vi "Mixed Mode Widget.vi"() -> ()   [LabVIEW 2009]
uses:
  lib/MixedMode/Messages/Target.ctl
  lib/Data Access Objects/Metadata/LBCB Number.ctl
  lib/MixedMode/Ramp Time Tuple.ctl
  lib/MixedMode Widget/Mixed Mode State Display.ctl
  lib/MixedMode/Mixed Mode States.ctl
  lib/MixedMode/Messages/Mixed Mode Command.ctl
  lib/MixedMode/Mixed Mode Command Action.ctl
  lib/MixedMode/Target Data.ctl
  lib/MixedMode Widget/Mixed Mode Widget Button States.ctl
  lib/MixedMode Widget/Target Pattern.ctl
  lib/MixedMode/Messages/Mixed Mode Status.ctl
  lib/MixedMode/Mixed Mode Covergance Status.ctl
  lib/MixedMode/Mixed Mode Cartesian Data.ctl
  lib/MixedMode Widget/NTCP MM Requests.ctl
  lib/MixedMode/MCL States.ctl
  lib/MixedMode Widget/Manual States.ctl
  lib/MixedMode Widget/Input File States.ctl
  lib/MixedMode Widget/NTCP Mixed Mode States.ctl
  lib/NTCP Client/NTCP 2 MM Message.ctl
  NTCP library/NTCP Commands.ctl
  lib/MixedMode/Messages/Mixed Mode Button Events Message.ctl
  lib/MixedMode/Messages/Mixed Mode Button Events.ctl
  lib/Apps/GUI Control.ctl
  lib/MixedMode/Messages/MM Widget Parameter Changes.ctl
  lib/MixedMode/Messages/Mixed Mode Gui Update Msg.ctl
  lib/MixedMode/Messages/Mixed Mode GUI Update Type.ctl
  lib/Global Data/Name Actions.ctl
  lib/MixedMode Widget/Blinkies.ctl
  lib/Apps/On Off Button.ctl
  lib/NTCP Client/MM 2 NTCP Message.ctl
  lib/Apps/Yes No Button.ctl
  lib/Apps/App Status Actions.ctl
  lib/Data Access Objects/Metadata/DAO Actions.ctl
  lib/MixedMode/Step DAO Actions.ctl
  lib/MixedMode Widget/Input File Step Actions.ctl
  lib/Launcher/NoPanelAppTypes.ctl
  lib/Launcher/Launcher Actions.ctl
  lib/Data Access Objects/Metadata/Persistant DAO Actions.ctl
  lib/MixedMode Widget/Skip NTCP Close Monitor.ctl
  lib/MixedMode Widget/Run Or Stop Result.ctl
panel:
  out "From Queue":string
  out "To Queue":string
  out "NTCP":T1
  out "MCL States":T5
  out "NTCP MM Requests":T6
  out "Force Limit":bool caption="Force"
  out "Displacement Limit":bool caption="Displacement"
  out "Messages":string
  out "Mixed Mode Status":T7={"LBCB Target"=[], "MixedModeStates"=enum."Idle", "LBCB Convergence"=[], "LBCB Measurements"=[]}
  in  "App Running":bool
  out "Button States":T12
  in  "App Stop":bool
  out "Mixed Mode Command":T13
  in  "Cartesian Type":bool caption="CartesianType"
  in  "Channel Data Tables":T16(tab)
  out "Cartesian Space Labels L1":string[](array[string])=["Commands (in/rad)", "Displacements (in/rad)", "Forces (lbs/lb*in)"]
  out "Cartesian Labels L1":string[](array[string])=["X", "Y", "Z", "Rx", "Ry", "Rz"]
  out "LBCB 1 Cartesian Space":dbl[][](array[numeric]) caption="LBCB 1"
  out "LBCB 2 Cartesian Space":dbl[][](array[numeric]) caption="LBCB 2"
  out "Cartesian Labels L2":string[](array[string])=["X", "Y", "Z", "Rx", "Ry", "Rz"]
  out "Cartesian Space Labels L2":string[](array[string])=["Commands (in/rad)", "Displacements (in/rad)", "Forces (lbs/lb*in)"]
  out "Actuator Space Labels L2":string[](array[string])=["Commands (in)", "Displacements (in)", "Forces (lbs)", "Integral"]
  out "Actuator Labels L2":string[](array[string])=["X1", "X2", "Y1", "Z1", "Z2", "Z3"]
  out "LBCB 2 Actuator Space":dbl[][](array[numeric]) caption="LBCB 2"
  out "LBCB 1 Actuator Space":dbl[][](array[numeric]) caption="LBCB 1"
  out "Actuator Labels L1":string[](array[string])=["X1", "X2", "Y1", "Z1", "Z2", "Z3"]
  out "Actuator Space Labels L1":string[](array[string])=["Commands (in)", "Displacements (in)", "Forces (lbs)", "Integral"]
  out "External Sensors":cluster{"Name":string, "Value":dbl}[](array[cluster])
  out "Test Statistics":cluster{"Steps":string, "Elapsed \nTime":dbl} {"Elapsed \nTime" format="%<%H:%M:%S>t"}
  in  "Mixed Mode Control Tabs":enum32{"Manual", "Input File", "NTCP"}(tab)
  in  "Set Initial Position":bool
  in  "Set Target":bool
  in  "Target Pattern":T17
  in  "Apply Pattern":bool
  out "Manual States":T18
  in  "Run Infile":bool
  out "Running":bool
  in  "Reset":bool
  in  "Load File":bool
  out "Input File States":T19
  in  "Connect Server":bool
  in  "Control Point":string="MDL-00-01"
  out "Connected":bool
  out "NTCP MM States":T20
  in  "Execute":cluster{"Auto":bool, "Start":bool, "Stop":bool}
  in  "Propose":T21
  out "Mixed Mode State Display":T22
  out "Current Values":T3[](array[typedef])
  in  "Ramp Times":cluster{"Displacement":T15, "Force":T15}={"Displacement"={"Ramp"=5.0, "Stab"=4.0, "Hold"=5.0}, "Force"={"Ramp"=5.0, "Stab"=4.0, "Hold"=5.0}}
  in  "Targets":T3[](array[typedef])
  # "Limit\nFaults"
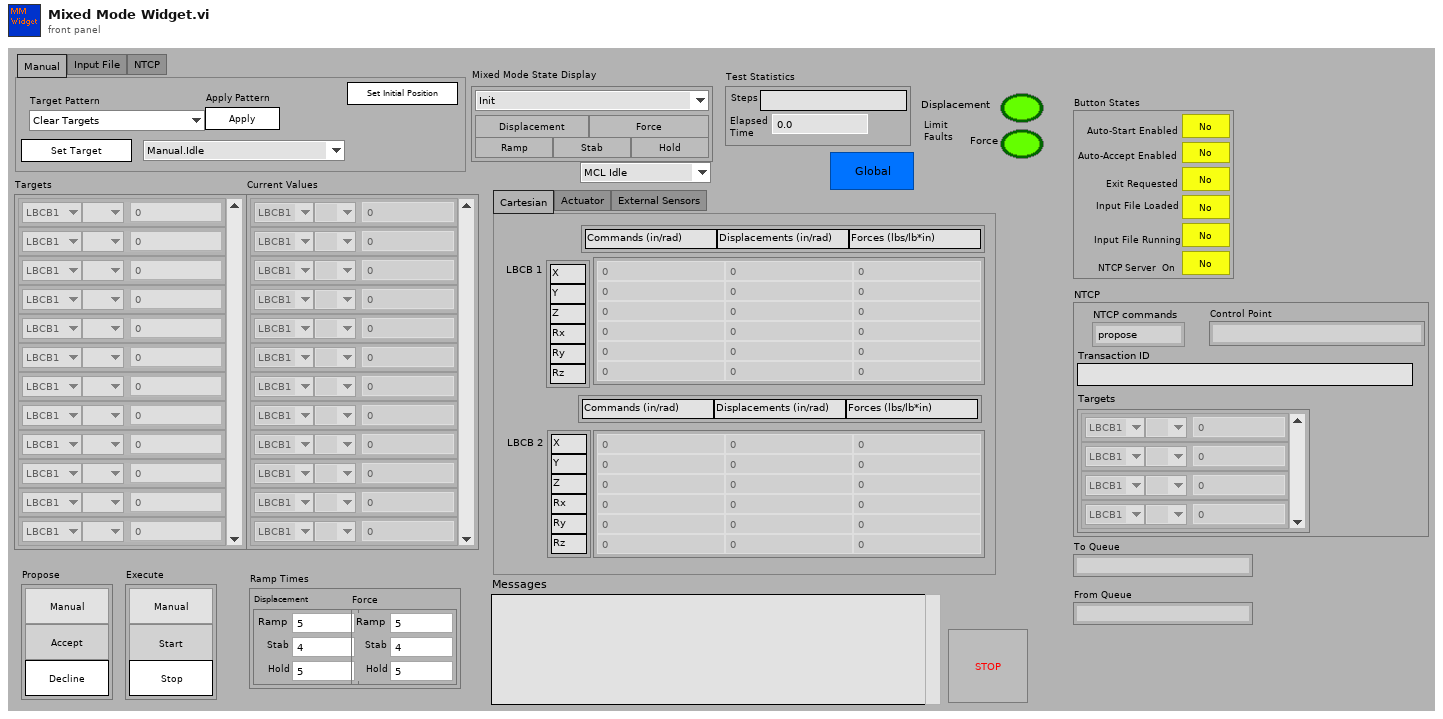
[diagram p1: front panel]
types:
  T1 = typedef "NTCP 2 MM Message.ctl" = cluster{"NTCP commands":T2, "Transaction ID":string, "Control Point":string, "Targets":T3[]}
  T2 = typedef "NTCP Commands.ctl" = enum16{"propose", "execute", "cancel", "set-parameter", "get-parameter", "open-session", "close-session", "get-control-point", "Unknown", "stop"}
  T3 = typedef "Target.ctl" = cluster{"LBCB Number":T4, "DOF Vectors":enum16{" ", "Dx", "Dy", "Dz", "Rx", "Ry", "Rz", "Fx", "Fy", "Fz", "Mx", "My", "Mz"}, "Amount":dbl}
  T4 = typedef "LBCB Number.ctl" = enum16{"LBCB1", "LBCB2"}
  T5 = typedef "MCL States.ctl" = enum16{"MCL Idle", "MCL Ramping", "MCL Holding", "MCL Aborting", "MCL Done", "MCL NOP"}
  T6 = typedef "NTCP MM Requests.ctl" = cluster{"Execute Pending":bool, "Propose Pending":bool, "Connected":bool, "Reset":bool}
  T7 = typedef "Mixed Mode Status.ctl" = cluster{"LBCB Target":T8[], "MixedModeStates":T9, "LBCB Convergence":T10[], "LBCB Measurements":T11[]}
  T8 = typedef "Target Data.ctl" = cluster{"Displacements":dbl[], "Command Type":enum16{"<None>", "Displacement", "Force"}[], "Forces":dbl[]}
  T9 = typedef "Mixed Mode States.ctl" = enum16{"Init", "Wait For DAQ", "Idle", "Start Initial Position", "Initial Position", "Start Initial Ramp", "Run Initial Ramp", "Start Iterative Stage", "Convergence Check", "Update Stiffness Jacobian", "Update Command", "Start Iterative Ramp", "Run Iterative Ramp", "Start Iterative Stabilize", "Iterative Stabilize", "Start Iterative Holding", "Iterative Holding", "Start Stabilize", "Stabilize", "Start Hold", "Holding", "Done", "Aborting", "Exit", "Nop"}
  T10 = typedef "Mixed Mode Covergance Status.ctl" = cluster{"IsConverged":bool[], "Force Errors":dbl[], "Controlling DOF":bool[]}
  T11 = typedef "Mixed Mode Cartesian Data.ctl" = cluster{"Displacements":dbl[], "Forces":dbl[]}
  T12 = typedef "Mixed Mode Widget Button States.ctl" = cluster{"Auto-Start Enabled":bool, "Auto-Accept Enabled":bool, "Exit Requested":bool, "Input File Loaded":bool, "Input File Running":bool, "NTCP Server  On":bool}
  T13 = typedef "Mixed Mode Command.ctl" = cluster{"Command":T14, "Ramp Times":cluster{"Initial":T15, "Iterative":T15}, "LBCB1":T8, "LBCB2":T8}
  T14 = typedef "Mixed Mode Command Action.ctl" = enum16{"Start Command", "Stop", "Exit", "No Op", "Start Acquisition", "Measure Initial Position"}
  T15 = typedef "Ramp Time Tuple.ctl" = cluster{"Ramp":dbl, "Stab":dbl, "Hold":dbl}
  T16 = enum32{"Cartesian", "Actuator", "External Sensors"}
  T17 = typedef "Target Pattern.ctl" = enum16{"Clear Targets", "Reset Targets to Zero", "Displacements Only", "Rotations Only", "Displacements & Rotations", "Forces Only", "Moments Only", "Forces & Moments"}
  T18 = typedef "Manual States.ctl" = enum16{"Manual.Idle", "Manual.WaitForStart", "Manual.WaitForMclRamp", "Manual.WaitForMclDone", "Manual.Abort", "Manual.InitialPosition"}
  T19 = typedef "Input File States.ctl" = enum16{"InputFile.Idle", "InputFile.WaitForRunning", "InputFile.StepsAvailable", "InputFile.LoadStep", "InputFile.WaitForAccept", "InputFile.WaitForStart", "InputFile.WaitForMclRamp", "InputFile.WaitForMclDone", "InputFile.StopRunning"}
  T20 = typedef "NTCP Mixed Mode States.ctl" = enum16{"Ntcp.Off", "Ntcp.WaitForProposal", "Ntcp.WaitForAccept", "Ntcp.WaitForExecute", "Ntcp.WaitForStart", "Ntcp.WaitForMclRamp", "Ntcp.WaitForMclDone", "Ntcp.Shutdown"}
  T21 = cluster{"Auto":bool, "Accept":bool, "Decline":bool}
  T22 = typedef "Mixed Mode State Display.ctl" = cluster{"MixedModeStates":T9, "Initial":bool, "Iterative":bool, "Ramp":bool, "Stab":bool, "Hold":bool}
  T23 = typedef "MM 2 NTCP Message.ctl" = cluster{"NTCP commands":T2, "Transaction ID":string, "Control Point":string, "Accepted":T24}
  T24 = typedef "Yes No Button.ctl" = bool
  T25 = typedef "Blinkies.ctl" = cluster{"Accept":T26, "Start":T26}
  T26 = typedef "On Off Button.ctl" = bool
  T27 = typedef "Name Actions.ctl" = enum16{"Init", "Get Names", "Get Index"}
  T28 = typedef "Mixed Mode Gui Update Msg.ctl" = cluster{"MM GUI Update Type":T29, "Targets":T3[], "State":bool, "Step":string}
  T29 = typedef "Mixed Mode GUI Update Type.ctl" = enum16{"Nop", "Targets", "Accept.Blink", "Start.Blink", "TestStats", "Control.Enabled", "StartTestTimer", "RunInputFile", "NTCP Server", "Propose.Auto", "Execute.Auto", "All Autos Off", "Input File Loaded", "Exit"}
  T30 = typedef "GUI Control.ctl" = cluster{"Command":T31, "LBCB Number":enum16{"LBCB1", "LBCB2"}}
  T31 = typedef "MM Widget Parameter Changes.ctl" = enum16{"Start", "Stop All", "Cartesian Type Changed", "Control Enabled", "Control Disabled", "NTCP Link On", "NTCP Link Off"}
  T32 = typedef "Mixed Mode Button Events Message.ctl" = cluster{"MM Control Events":T33, "Button States":T12}
  T33 = typedef "Mixed Mode Button Events.ctl" = enum16{"Propose.Accept", "Propose.Decline", "Execute.Start", "Execute.Stop", "TargetSet", "InputFile.Load", "InputFile.Reset", "InputFile.Pause", "InputFile.Run", "CartesianType.Changed", "NCTP.ConnectToServer", "NTCP.DisconnectFromServer", "Application.Stop", "Control.Enabled", "Control.Disabled", "ControlType.Changed", "Nop", "Manual.SetInitialPosition"}
  T34 = typedef "DAO Actions.ctl" = enum16{"Init", "Get", "Set"}
  T35 = typedef "App Status Actions.ctl" = enum16{"Init", "Get Status", "Running", "Control", "Autobalanced", "Data Acquisition", "Set App State", "DAQ Started", "Set LBCB State", "Set All", "Set Cont Logging", "Set Step Logging", "Set MM Logging", "Set Volt Logging", "Set Cart Type", "Set DAQ Link", "Set NTCP Link"}
  T36 = typedef "Step DAO Actions.ctl" = enum16{"Init", "Set", "Get", "Reset Count"}
  T37 = typedef "App Status.ctl" = cluster{"Running":bool, "Controlling L2":bool, "Autobalance L2":bool, "Data Acquisition":bool, " App State":T38, "DAQ Started":bool, "LBCB 1 State":T39, "LBCB 2 State":T39, "Controlling L1":bool, "Autobalance L1":bool, "Cartesian Type":bool, "Continuous Logging":bool, "Step Logging":bool, "Voltage Logging":bool, "Mixed Mode Logging":bool, "DAQ Link":bool, "NTCP Link ":bool}
  T38 = typedef "AppStates.ctl" = enum16{"Starting OM", "Initializing Displays", "Setting up Archiving", "Setting Up DAQ Channels", "Start DAQ", "DAQ Starting", "Controlling LBCBs", "Stopping OM"}
  T39 = typedef "Lbcb Control Loop States.ctl" = enum16{"Idle", "Start Selected", "Load Last Command", "Start Autobalancing", "Autobalancing", "Control Loop Initialized", "Control Enabled"}
  T40 = enum8{"Enabled", "Disabled", "Disabled and Grayed Out"}
  T41 = typedef "Input File Step Actions.ctl" = enum16{"Load", "Next Step", "Reset", "Get Step", "Backup"}
  T42 = typedef "Run Or Stop Result.ctl" = enum16{"Nevermind", "Run", "Stop"}
  T43 = typedef "Load Step.ctl" = cluster{"Step Number":u32, "Targets":T3[]}
  T44 = typedef "Accepted or Declined.ctl" = enum16{"No Decision Yet", "Accepted", "Declined", "Abort"}
  T45 = typedef "Stop Requests.ctl" = enum16{"Nothing", "Stop Requested", "Abort Requested"}
  T46 = typedef "MCL Done Or Abort.ctl" = enum16{"Done", "Abort", "Still Running"}
  T47 = typedef "NoPanelAppTypes.ctl" = enum16{"NTCP Socket", "Data Archiving", "DAQ Link", "Control Loops", "Autobalance Monitor", "Mixed Mode Monitor", "Cmd Disp Diffs"}
  T48 = typedef "Launcher Actions.ctl" = enum16{"Launch", "Stop All", "Stop", "Kill", "Running?", "Init"}
  T49 = typedef "Persistant DAO Actions.ctl" = enum16{"Init", "Get", "Set", "Load", "Save"}
  T50 = typedef "Skip NTCP Close Monitor.ctl" = enum16{"Skip Nothing", "Skip NTCP", "Skip Button Event"}
  T51 = typedef "Network Parameters.ctl" = cluster{"Port Number":u16, "Notification Name":string, "Wait For Notification Timeout":i32}
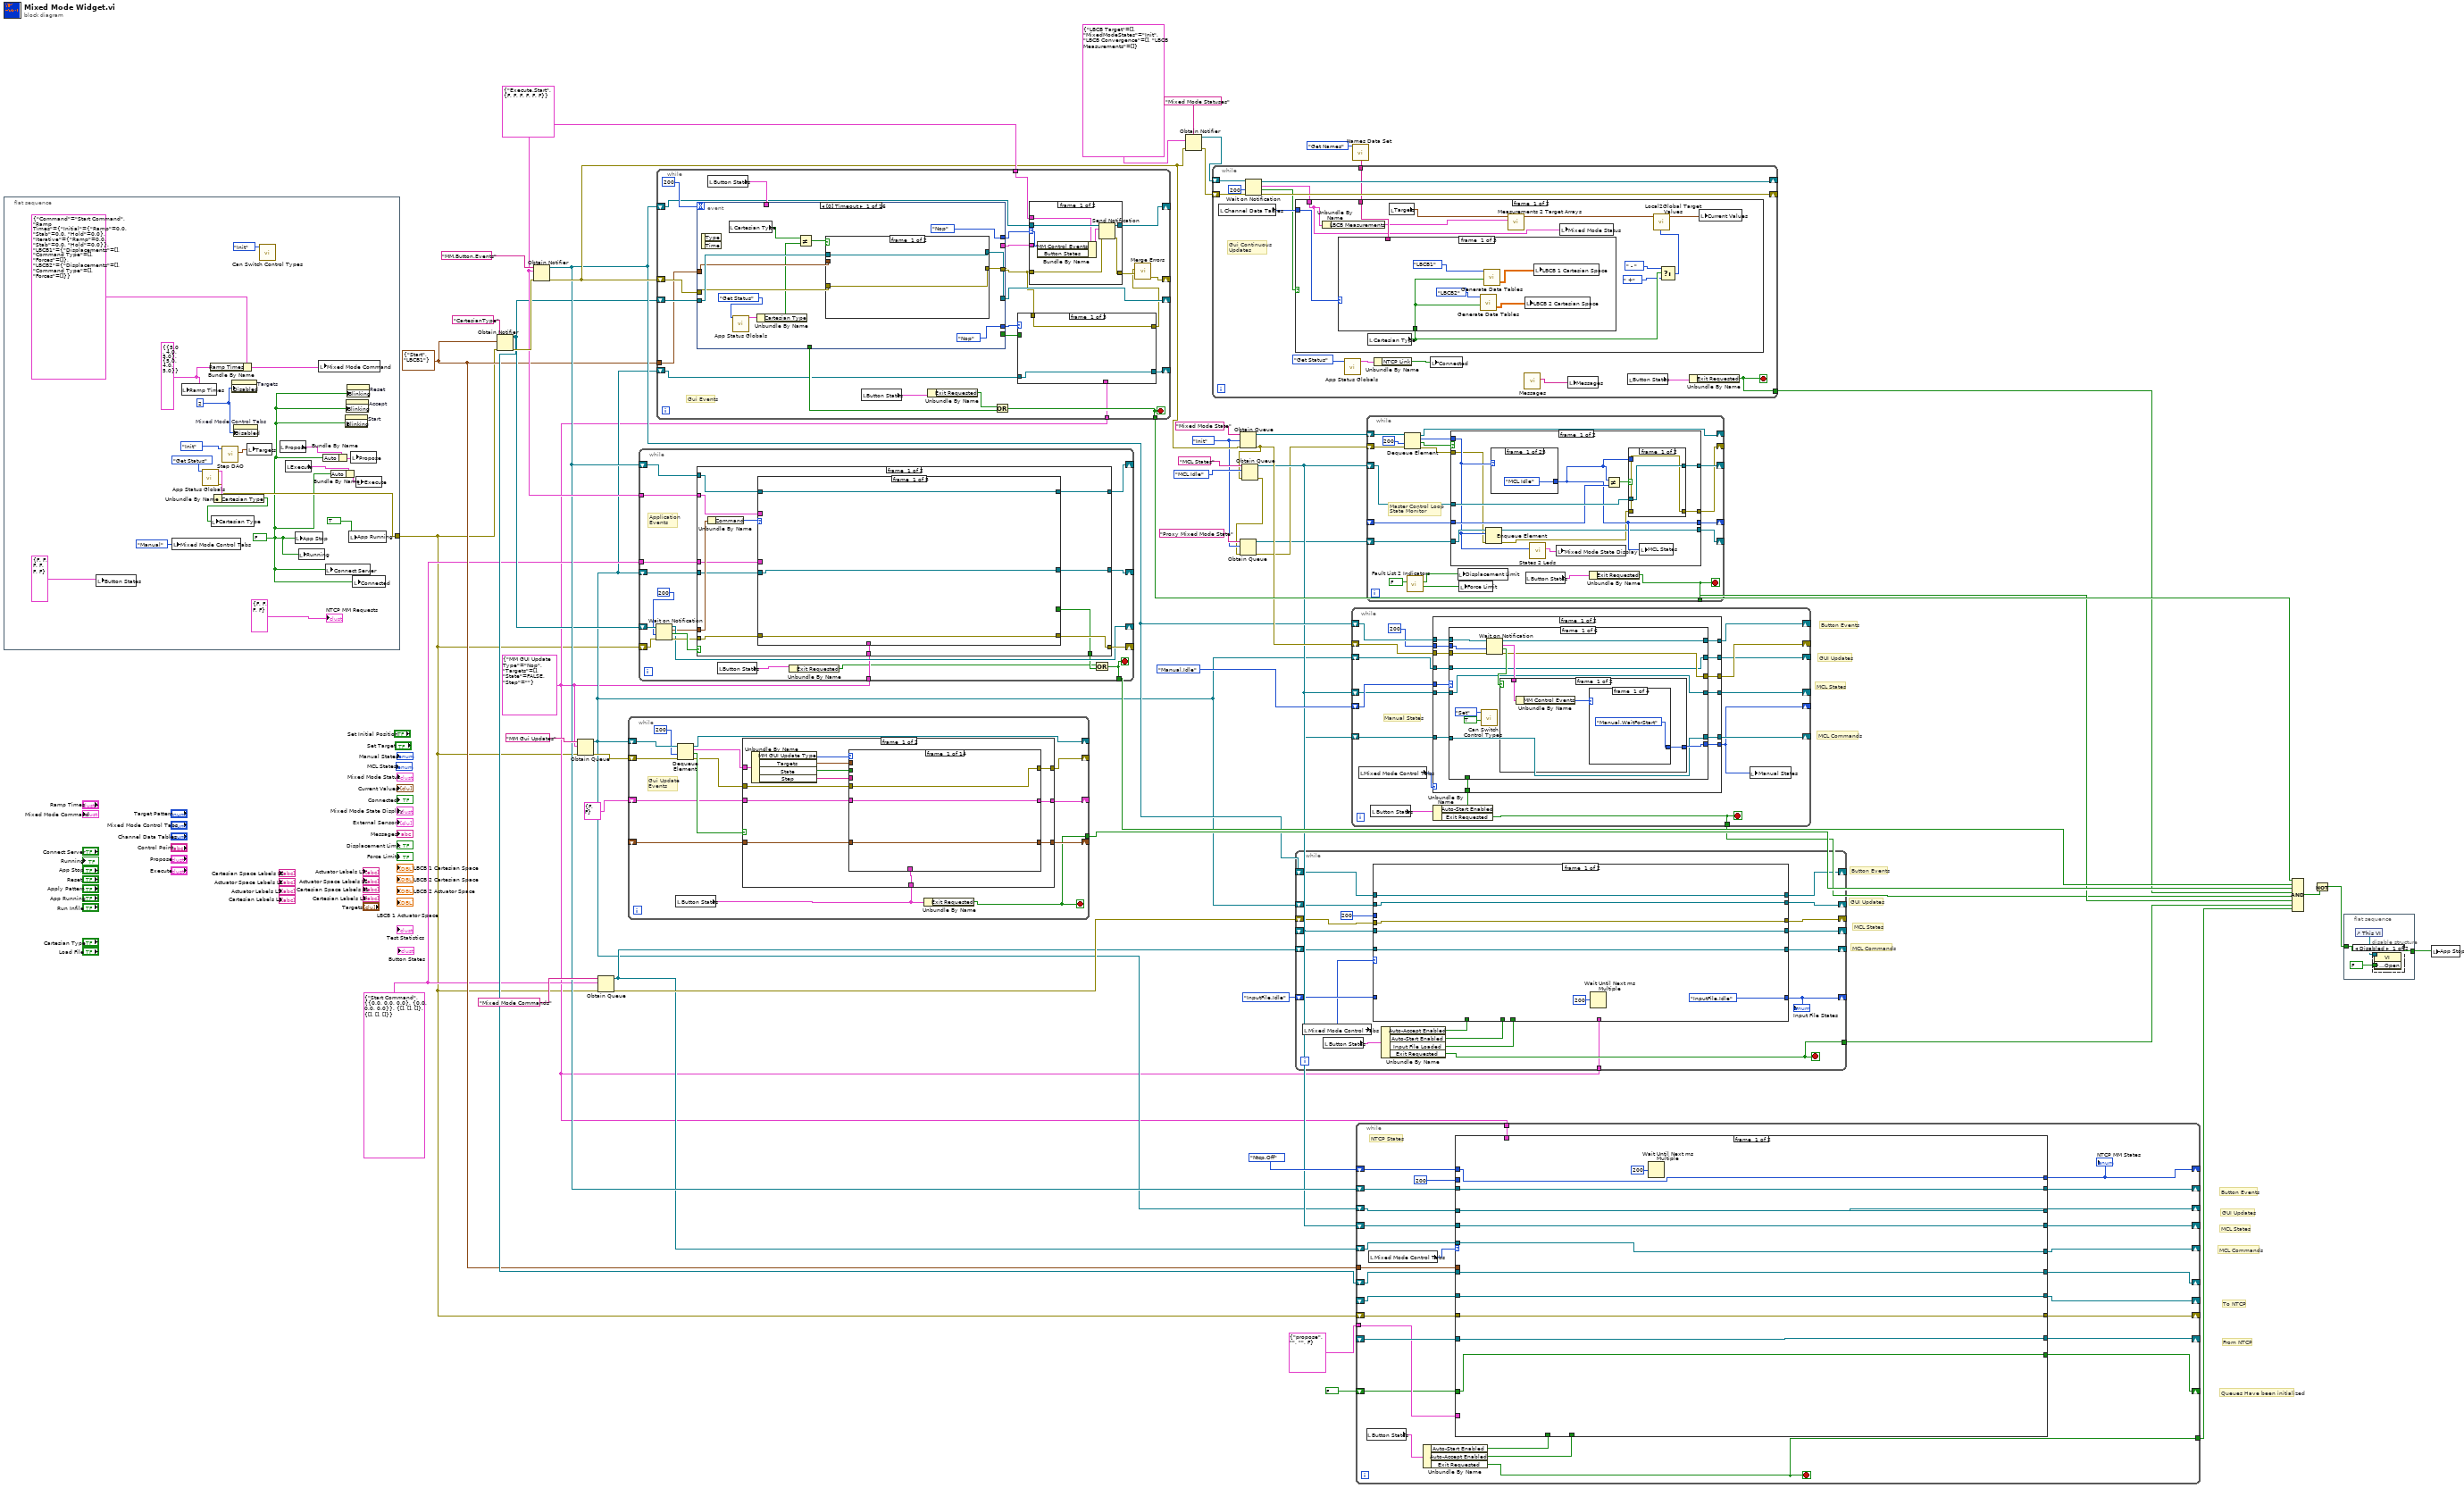
[diagram p0: block diagram]
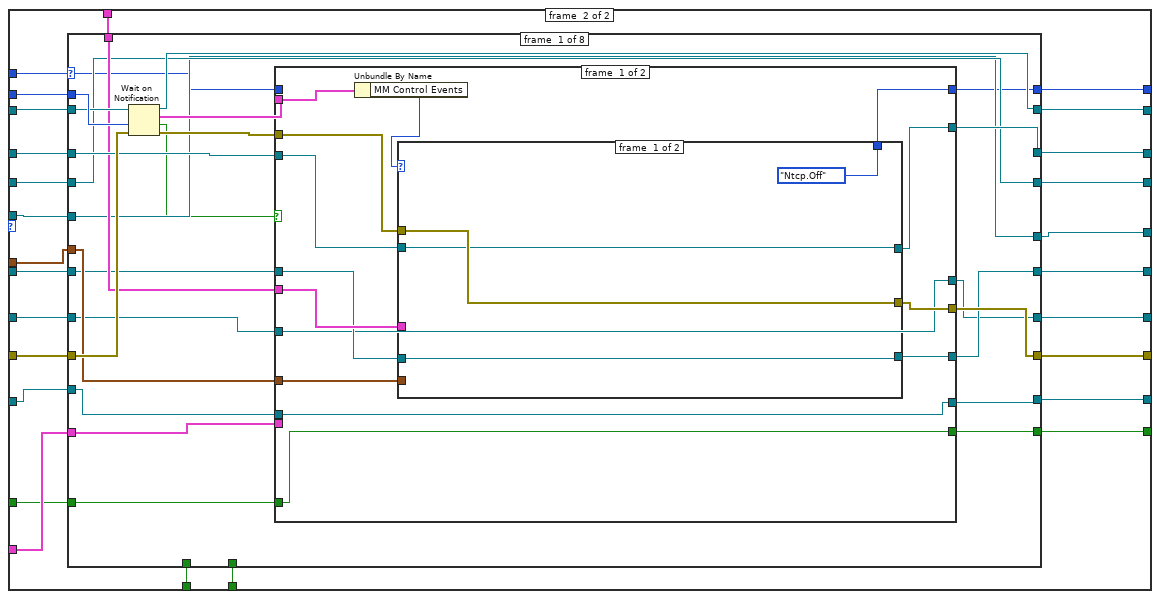
[diagram p2: hidden frame]
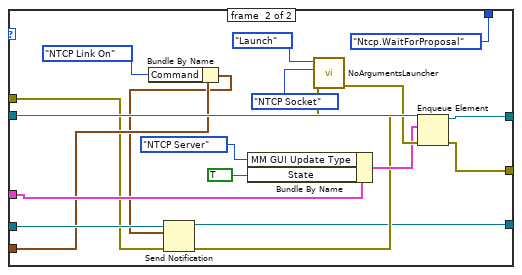
[diagram p3: hidden frame]
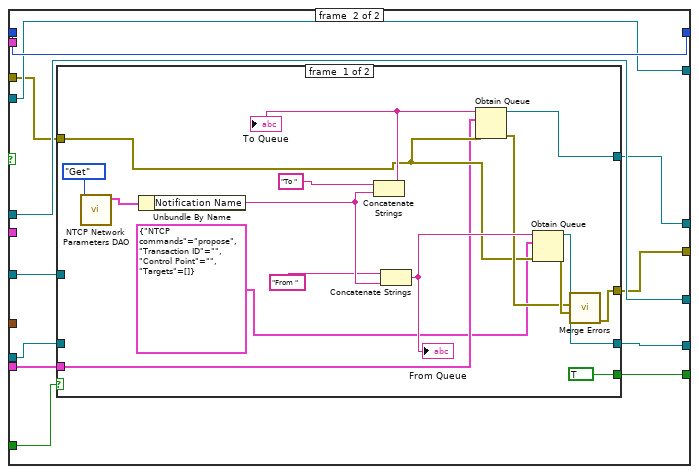
[diagram p4: hidden frame]
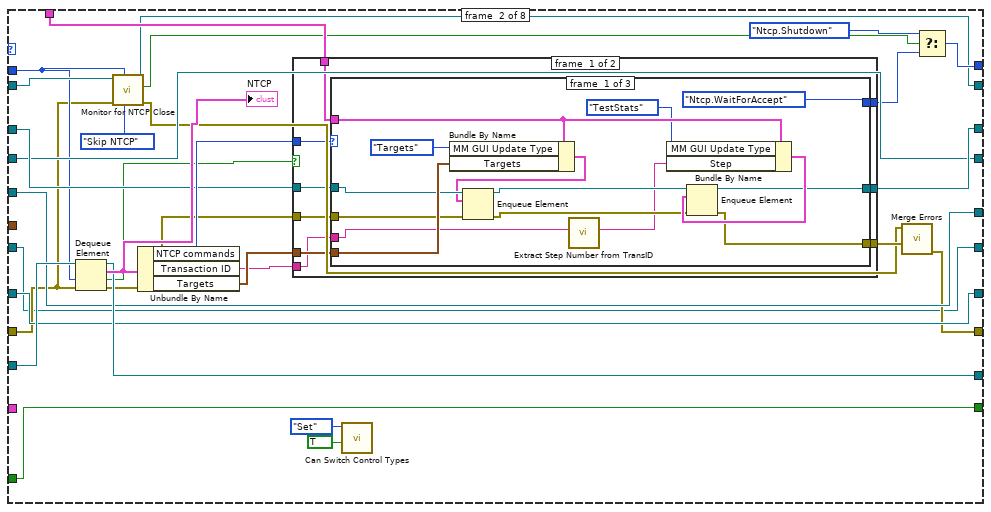
[diagram p6: hidden frame]
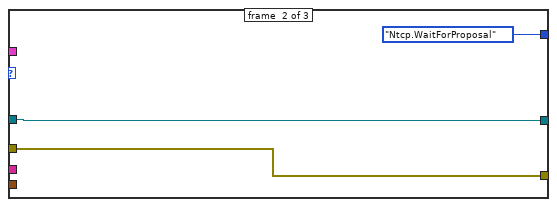
[diagram p7: hidden frame]
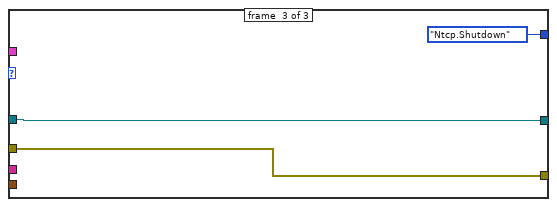
[diagram p8: hidden frame]
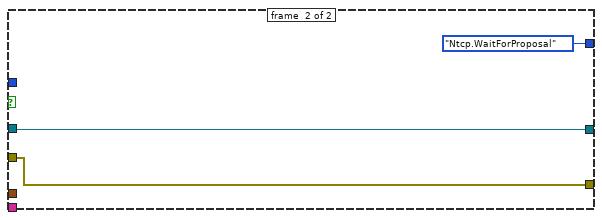
[diagram p9: hidden frame]
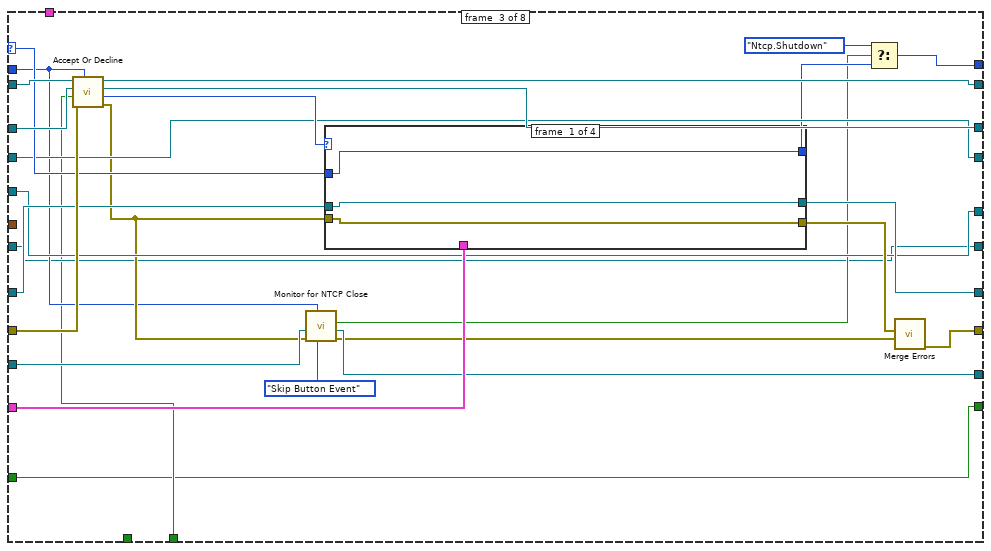
[diagram p10: hidden frame]
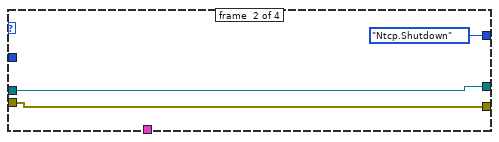
[diagram p11: hidden frame]
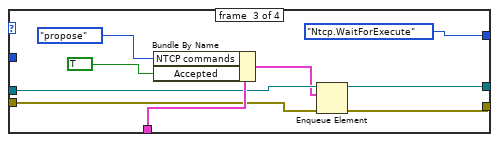
[diagram p12: hidden frame]
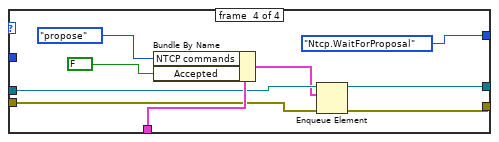
[diagram p13: hidden frame]
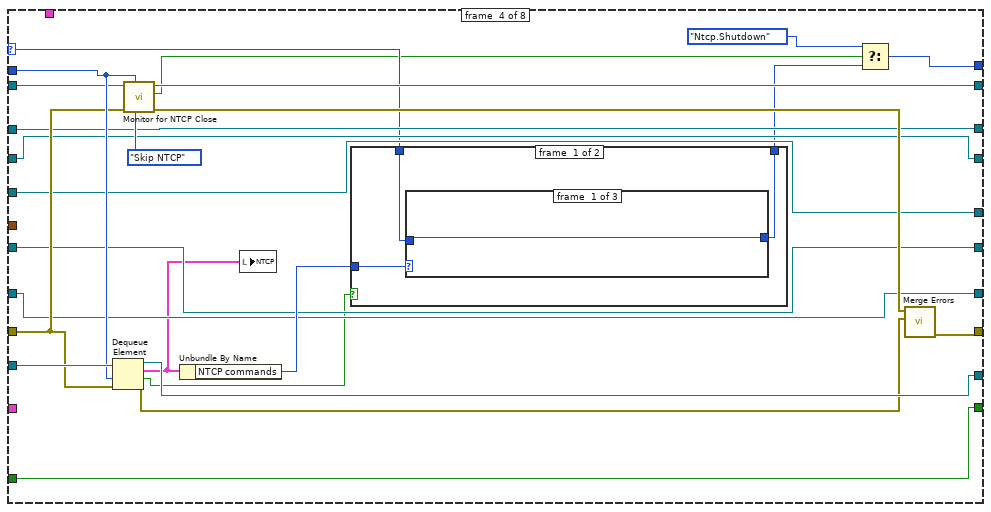
[diagram p14: hidden frame]
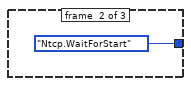
[diagram p15: hidden frame]
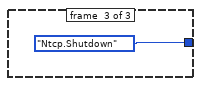
[diagram p16: hidden frame]
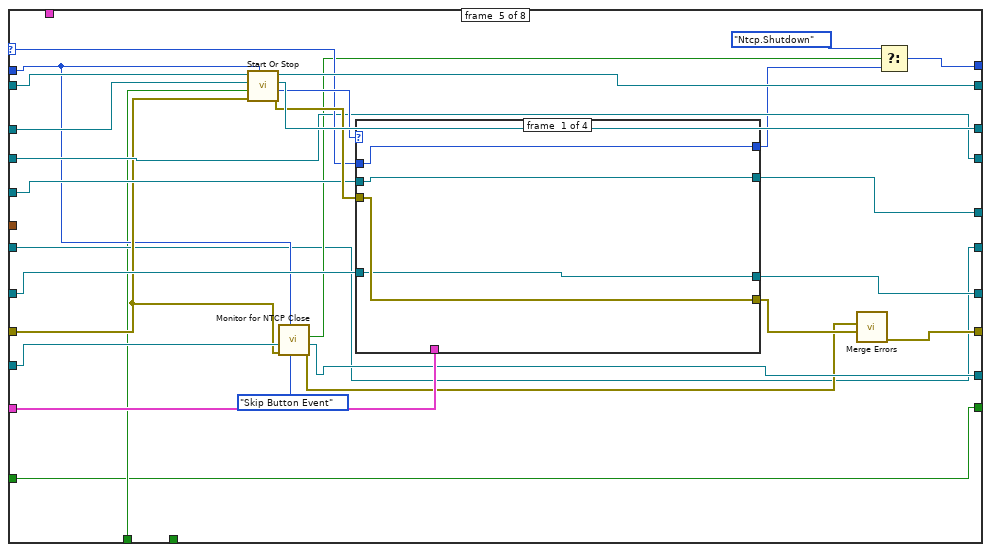
[diagram p18: hidden frame]
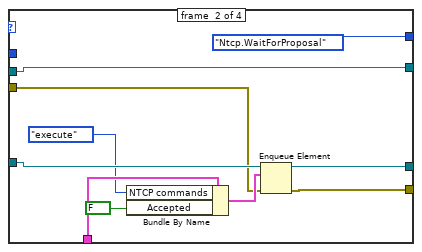
[diagram p19: hidden frame]
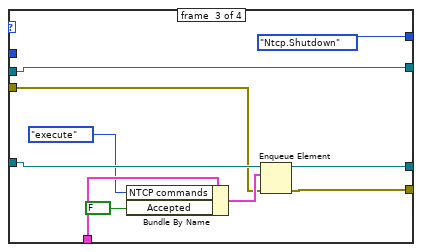
[diagram p20: hidden frame]
diagram:
  w12 = T13 {"Command"=enum."Start Command", "Ramp Times"={"Initial"={"Ramp"=0.0, "Stab"=0.0, "Hold"=0.0}, "Iterative"={"Ramp"=0.0, "Stab"=0.0, "Hold"=0.0}}, "LBCB1"={"Displacements"=[], "Command Type"=[], "Forces"=[]}, "LBCB2"={"Displacements"=[], "Command Type"=[], "Forces"=[]}} ("Mixed Mode Command In")
  w4 = Mixed_Mode_States."Init" ("f")
  w9 = T28 {"MM GUI Update Type"=enum."Nop", "Targets"=[], "State"=FALSE, "Step"=""} ("MM Gui Update Msg")
  w14 = T30 {"Command"=enum."Start", "LBCB Number"=enum."LBCB1"} ("GUI Control")
  w45 = T32 {"MM Control Events"=enum."Execute.Start", "Button States"={"Auto-Start Enabled"=FALSE, "Auto-Accept Enabled"=FALSE, "Exit Requested"=FALSE, "Input File Loaded"=FALSE, "Input File Running"=FALSE, "NTCP Server  On"=FALSE}} ("MM Button Events Msg")
  # "Queues Have been initialized"
  # "Button Events"
  # "GUI Updates"
  # "MCL States"
  # "MCL Commands"
  # "From NTCP"
  # "To NTCP"
  # "Button Events"
  # "GUI Updates"
  # "MCL States"
  # "MCL Commands"
  # "Button Events"
  # "GUI Updates"
  # "MCL States"
  # "MCL Commands"
  n1 = flat-sequence {
    tunnel: [w69] -> w8
    frame #0 {
      w58 = cluster{"Initial":T15, "Iterative":T15} {"Initial"={"Ramp"=5.0, "Stab"=4.0, "Hold"=5.0}, "Iterative"={"Ramp"=5.0, "Stab"=4.0, "Hold"=5.0}} ("Ramp Times")
      w59 = u8 2 ("Disabled")
      w53 = FALSE ("Exit")
      n2 = local write "Button States"(T12 {"Auto-Start Enabled"=FALSE, "Auto-Accept Enabled"=FALSE, "Exit Requested"=FALSE, "Input File Loaded"=FALSE, "Input File Running"=FALSE, "NTCP Server  On"=FALSE} ("Mixed Mode Widget Requests")) -> ()
      n3 = local write "Mixed Mode Control Tabs"(enum32{"Manual", "Input File", "NTCP"}."Manual" ("Mixed Mode Control Tabs")) -> ()
      n4 = local write "Ramp Times"(w58) -> ()
      n5 = call "App Status Globals.vi"("App Status Actions"=App_Status_Actions."Get Status") -> ("App Status Out"=w71:T37, "error out"=w69:errorcluster)  [unwired: 5 in, 8 out]
      n6 = Bundle By Name(cluster=T13 {"Command"=enum."Start Command", "Ramp Times"={"Initial"={"Ramp"=0.0, "Stab"=0.0, "Hold"=0.0}, "Iterative"={"Ramp"=0.0, "Stab"=0.0, "Hold"=0.0}}, "LBCB1"={"Displacements"=[], "Command Type"=[], "Forces"=[]}, "LBCB2"={"Displacements"=[], "Command Type"=[], "Forces"=[]}} ("Mixed Mode Command"), "Ramp Times"=w58) -> (w56:T13)
      n7 = Unbundle By Name(w71) -> ("Cartesian Type"=w70:bool)
      n8 = local write "Cartesian Type"(w70) -> ()
      n9 = call "Step DAO.vi"("Step DAO Actions"=Step_DAO_Actions."Init") -> ("Step Out"=w67:T3[])  [unwired: 3 in, 7 out]
      n10 = property on="Targets" class="Arr (strict)"("Disabled"=w59) -> ()  [unwired: 2 in, 2 out]
      n11 = property on="Mixed Mode Control Tabs" class="TabCtl (strict)"("Disabled"=w59) -> ()  [unwired: 2 in, 2 out]
      n12 = local write "Targets"(w67) -> ()
      n13 = call "Can Switch Control Types.vi"("DAO Actions"=DAO_Actions."Init") -> ()  [unwired: 10 in, 1 out]
      n14 = local read "Propose"() -> (w63:T21)
      n15 = local read "Execute"() -> (w61:cluster{"Auto":bool, "Start":bool, "Stop":bool})
      n16 = local write "App Stop"(w53) -> ()
      n17 = local write "Running"(w53) -> ()
      n18 = local write "Mixed Mode Command"(w56) -> ()
      n19 = Bundle By Name(cluster=w63, "Auto"=w53) -> (w64:T21)
      n20 = local write "Connect Server"(w53) -> ()
      n21 = Bundle By Name(cluster=w61, "Auto"=w53) -> (w62:cluster{"Auto":bool, "Start":bool, "Stop":bool})
      n22 = property on="Start" class="Bool (strict)"("Blinking"=w53) -> ()  [unwired: 2 in, 2 out]
      n23 = property on="Accept" class="Bool (strict)"("Blinking"=w53) -> ()  [unwired: 2 in, 2 out]
      n24 = property on="Reset" class="Bool"("Blinking"=w53) -> ()  [unwired: 2 in, 2 out]
      n25 = local write "App Running"(TRUE) -> ()
      n26 = local write "Propose"(w64) -> ()
      n27 = local write "Connected"(w53) -> ()
      n28 = local write "Execute"(w62) -> ()
      "NTCP MM Requests" <- T6 {"Execute Pending"=FALSE, "Propose Pending"=FALSE, "Connected"=FALSE, "Reset"=FALSE} ("NTCP MM Requests")
    }
  }
  n29 = Obtain Notifier(name (unnamed)="CartesianType", notification data type=w14, error in (no error)=w8) -> (notifier out=w15:refnum<notifier>, error out=w46:errorcluster)  [unwired: 1 in, 1 out]
  n30 = Obtain Notifier(name (unnamed)="MM.Button.Events", notification data type=w45, error in (no error)=w46) -> (notifier out=w18:refnum<notifier>, error out=w31:errorcluster)  [unwired: 1 in, 1 out]
  n31 = Obtain Queue(name (unnamed)="MM Gui Updates", element data type=w9, error in (no error)=w8) -> (queue out=w11:refnum<queue>, error out=w41:errorcluster)  [unwired: 2 in, 1 out]
  n32 = Obtain Queue(name (unnamed)="Mixed Mode Commands", element data type=w12, error in (no error)=w8) -> (queue out=w13:refnum<queue>, error out=w20:errorcluster)  [unwired: 2 in, 1 out]
  n33 = while {
    shift-right: [w78] -> _
    shift-left: w41 -> [w83]
    shift-right: [w82] -> _
    shift-left: w11 -> [w85]
    shift-right: [w77] -> _
    shift-left: _ -> [w76]
    tunnel: [w75] -> w40
    shift-right: [w72] -> _
    shift-left: T25 {"Accept"=FALSE, "Start"=FALSE} ("Blinkies") -> [w73]
    stop <- w75 stop-if-true
    # "Gui Update\nEvents"
    n34 = local read "Button States"() -> (w74:T12)
    n35 = Dequeue Element(queue=w85, timeout in ms (-1)=200, error in (no error)=w83) -> (queue out=w82:refnum<queue>, element=w81:T28, timed out?=w80:bool, error out=w79:errorcluster)
    n36 = case shown="True" w80 {
      tunnel: w81 -> [w97 _]
      tunnel: w79 -> [w93 w194]
      tunnel: [w92 w194] -> w78
      tunnel: [w90 w193] -> w77
      tunnel: w76 -> [w89 w193]
      tunnel: w74 -> [w88 _]
      tunnel: w73 -> [w87 w192]
      tunnel: [w86 w192] -> w72
      frame #0 {
        n37 = Unbundle By Name(w97) -> ("MM GUI Update Type"=w96:T29, "Targets"=w95:T3[], "State"=w94:bool, "Step"=w91:string)
        n38 = case shown="\"Exit\"" w96 {
          tunnel: w95 -> [_ _ w107 _ _ _ _ _ _ _ _ _ _ _]
          tunnel: w94 -> [_ _ _ w109 w121 _ w141 w147 w154 _ w170 w175 w184 _]
          tunnel: w93 -> [w100 w103 w105 w115 w127 w133 w145 w151 w157 w163 w168 w174 w182 w190]
          tunnel: [w100 w103 w105 w114 w126 w133 w145 w151 w157 w163 w166 w174 w182 w190] -> w92
          tunnel: w91 -> [_ _ _ _ _ w137 _ _ _ _ _ _ _ _]
          tunnel: [w99 w102 w106 w113 w125 w134 w143 w149 w152 w159 w165 w179 w187 w191] -> w90
          tunnel: w89 -> [w99 w102 w106 w113 w125 w134 _ _ w152 w159 w165 w179 w187 _]
          tunnel: w88 -> [_ _ _ _ _ _ w142 w148 w155 w161 _ w178 w186 _]
          tunnel: w87 -> [w98 w101 w104 w110 w122 w132 w144 w150 w156 w162 w164 w173 w181 w189]
          tunnel: [w98 w101 w104 w108 w120 w132 w144 w150 w156 w162 w164 w173 w181 w189] -> w86
          frame #0 {
          }
          frame #1 {
          }
          frame #2 {
            n39 = local write "Targets"(w107) -> ()
          }
          frame #3 {
            n40 = Unbundle By Name(w110) -> ("Start"=w111:T26)
            n41 = Not Equal?(x=w109, y=w111) -> (x != y?=w112:T26)
            n42 = case shown="False" w112 {
              tunnel: w115 -> [w116 w119]
              tunnel: w109 -> [_ w118]
              tunnel: [w116 w117] -> w114
              frame #0 {
              }
              frame #1 {
                n43 = property on="Start" class="Bool (strict)"(error in=w119, "Blinking"=w118) -> (error out=w117:errorcluster)  [unwired: 1 in, 1 out]
              }
            }
            n44 = Bundle By Name(cluster=w110, "Start"=w109) -> (w108:T25)
          }
          frame #4 {
            n45 = Unbundle By Name(w122) -> ("Accept"=w123:T26)
            n46 = Not Equal?(x=w121, y=w123) -> (x != y?=w124:T26)
            n47 = case shown="True" w124 {
              tunnel: w127 -> [w128 w131]
              tunnel: w121 -> [_ w130]
              tunnel: [w128 w129] -> w126
              frame #0 {
              }
              frame #1 {
                n48 = property on="Accept" class="Bool (strict)"(error in=w131, "Blinking"=w130) -> (error out=w129:errorcluster)  [unwired: 1 in, 1 out]
              }
            }
            n49 = Bundle By Name(cluster=w122, "Accept"=w121) -> (w120:T25)
          }
          frame #5 {
            n50 = Get Date/Time In Seconds() -> (seconds since 1Jan1904=w135:timestamp)
            n51 = Subtract(x=w135, y=w134) -> (x-y=w136:dbl)
            n52 = Bundle By Name(cluster=cluster{"Steps":string, "Elapsed \nTime":dbl} {"Steps"="", "Elapsed \nTime"=0.0} ("Test Statistics"), "Steps"=w137, "Elapsed \nTime"=w136) -> (w138:cluster{"Steps":string, "Elapsed \nTime":dbl})
            n53 = local write "Test Statistics"(w138) -> ()
          }
          frame #6 {
            n54 = Bundle By Name(cluster=w142, "Input File Running"=w141) -> (w140:T12)
            n55 = local write "Running"(w141) -> ()
            n56 = local write "Button States"(w140) -> ()
            n57 = Get Date/Time In Seconds() -> (seconds since 1Jan1904=w143:timestamp)
          }
          frame #7 {
            n58 = Bundle By Name(cluster=w148, "NTCP Server  On"=w147) -> (w146:T12)
            n59 = local write "Connect Server"(w147) -> ()
            n60 = local write "Button States"(w146) -> ()
            n61 = Get Date/Time In Seconds() -> (seconds since 1Jan1904=w149:timestamp)
          }
          frame #8 {
            n62 = Bundle By Name(cluster=w155, "Input File Loaded"=w154) -> (w153:T12)
            n63 = local write "Button States"(w153) -> ()
          }
          frame #9 {
            n64 = Bundle By Name(cluster=w161, "Exit Requested"=TRUE) -> (w160:T12)
            n65 = local write "Button States"(w160) -> ()
          }
          frame #10 {
            n66 = Select(t=T40."Enabled" ("Disabled"), s=w170, f=T40."Disabled and Grayed Out" ("Disabled")) -> (s? t:f=w169:T40)
            n67 = property on="Mixed Mode Control Tabs" class="TabCtl (strict)"(error in=w168, "DisabledEnum"=w169) -> (error out=w167:errorcluster)  [unwired: 1 in, 1 out]
            n68 = property on="Targets" class="Arr (strict)"(error in=w167, "DisabledEnum"=w169) -> (error out=w166:errorcluster)  [unwired: 1 in, 1 out]
          }
          frame #11 {
            n69 = Bundle By Name(cluster=w178, "Auto-Accept Enabled"=w175) -> (w177:T12)
            n70 = Bundle By Name(cluster=T21 {"Auto"=FALSE, "Accept"=FALSE, "Decline"=FALSE} ("Propose"), "Auto"=w175) -> (w176:T21)
            n71 = local write "Button States"(w177) -> ()
            n72 = local write "Propose"(w176) -> ()
          }
          frame #12 {
            n73 = Bundle By Name(cluster=w186, "Auto-Start Enabled"=w184) -> (w185:T12)
            n74 = Bundle By Name(cluster=T21 {"Auto"=FALSE, "Accept"=FALSE, "Decline"=FALSE} ("Propose"), "Auto"=w184) -> (w183:T21)
            n75 = local write "Button States"(w185) -> ()
            n76 = local write "Execute"(w183) -> ()
          }
          frame #13 {
            n77 = Get Date/Time In Seconds() -> (seconds since 1Jan1904=w191:timestamp)
          }
        }
      }
      frame #1 {
      }
    }
    n78 = Unbundle By Name(w74) -> ("Exit Requested"=w75:bool)
  }
  n79 = while {
    shift-right: [w203] -> _
    shift-left: w18 -> [w205]
    shift-right: [w208] -> _
    shift-left: w15 -> [w212]
    shift-right: [w209] -> _
    shift-left: w8 -> [w211]
    tunnel: w45 -> [w204]
    tunnel: [w197] -> w43
    shift-right: [w199] -> _
    shift-left: w11 -> [w201]
    tunnel: w9 -> [w200]
    tunnel: w12 -> [w195]
    stop <- w197 stop-if-true
    # "Application\nEvents"
    n80 = Wait on Notification(notifier=w212, timeout in ms (-1)=200, error in (no error)=w211) -> (notifier out=w208:refnum<notifier>, notification=w207:T30, timed out?=w213:bool, error out=w210:errorcluster)  [unwired: 1 in]
    n81 = case shown="True" w213 {
      tunnel: w210 -> [w220 w285]
      tunnel: [w219 w285] -> w209
      tunnel: w207 -> [w225 _]
      tunnel: w205 -> [w222 w284]
      tunnel: w204 -> [w223 _]
      tunnel: [w221 w284] -> w203
      tunnel: [w218 _] -> w202
      tunnel: w201 -> [w217 w283]
      tunnel: w200 -> [w216 _]
      tunnel: [w215 w283] -> w199
      tunnel: w195 -> [w214 _]
      frame #0 {
        n82 = Unbundle By Name(w225) -> ("Command"=w224:T31)
        n83 = case shown="\"Control Enabled\"" w224 {
          tunnel: w223 -> [_ w242 w260 w274 w282]
          tunnel: w222 -> [w228 w237 w256 w269 w276]
          tunnel: [w228 w238 w257 w270 w277] -> w221
          tunnel: w220 -> [w227 w239 w248 w261 w279]
          tunnel: [w227 w234 w244 w271 w278] -> w219
          tunnel: [_ w236 _ _ _] -> w218
          tunnel: w217 -> [w226 w232 w249 w268 w275]
          tunnel: w216 -> [_ w231 _ w265 _]
          tunnel: [w226 w233 w243 w267 w275] -> w215
          tunnel: w214 -> [_ _ _ _ _]
          frame #0 {
          }
          frame #1 {
            w236 = TRUE ("Button States.Exit Requested")
            n84 = Bundle By Name(cluster=w242, "MM Control Events"=Mixed_Mode_Button_Events."Application.Stop", "Button States.Exit Requested"=w236) -> (w240:T32)
            n85 = Bundle By Name(cluster=w231, "MM GUI Update Type"=Mixed_Mode_GUI_Update_Type."Exit") -> (w230:T28)
            n86 = Send Notification(notification=w240, notifier=w237, error in (no error)=w239) -> (notifier out=w238:refnum<notifier>, error out=w235:errorcluster)
            n87 = Enqueue Element(queue=w232, element=w230, error in (no error)=w235) -> (queue out=w233:refnum<queue>, error out=w234:errorcluster)  [unwired: 1 in, 1 out]
          }
          frame #2 {
            n88 = local read "Targets"() -> (w255:T3[])
            n89 = call "App Status Globals.vi"("App Status Actions"=App_Status_Actions."Get Status") -> ("App Status Out"=w253:T37)  [unwired: 5 in, 9 out]
            n90 = Unbundle By Name(w253) -> ("Cartesian Type"=w246:bool)
            n91 = Select(t=enum16{" +", " - "}." - " ("Direction"), s=w246, f=enum16{" +", " - "}." +") -> (s? t:f=w251:enum16{" +", " - "})
            n92 = call "Local2Global Target Values.vi"("Direction"=w251, "Target  Inputs"=w255) -> ("Target  Outputs"=w247:T3[])  [unwired: 9 in]
            n93 = local write "Cartesian Type"(w246) -> ()
            n94 = Bundle By Name(cluster=w260, "MM Control Events"=Mixed_Mode_Button_Events."CartesianType.Changed") -> (w258:T32)
            n95 = call "Autos Off.vi"("error in"=w248, "Targets"=w247, "queue in"=w249) -> ("error out"=w245:errorcluster, "queue out"=w243:refnum<queue>)  [unwired: 1 in]
            n96 = Send Notification(notification=w258, notifier=w256, error in (no error)=w245) -> (notifier out=w257:refnum<notifier>, error out=w244:errorcluster)
          }
          frame #3 {
            n97 = Bundle By Name(cluster=w265, "MM GUI Update Type"=Mixed_Mode_GUI_Update_Type."Control.Enabled", "State"=TRUE) -> (w262:T28)
            n98 = Bundle By Name(cluster=w274, "MM Control Events"=Mixed_Mode_Button_Events."Control.Enabled") -> (w272:T32)
            n99 = Enqueue Element(queue=w268, element=w262, error in (no error)=w261) -> (queue out=w267:refnum<queue>, error out=w266:errorcluster)  [unwired: 1 in, 1 out]
            n100 = Send Notification(notification=w272, notifier=w269, error in (no error)=w266) -> (notifier out=w270:refnum<notifier>, error out=w271:errorcluster)
          }
          frame #4 {
            n101 = Bundle By Name(cluster=w282, "MM Control Events"=Mixed_Mode_Button_Events."Control.Disabled") -> (w280:T32)
            n102 = Send Notification(notification=w280, notifier=w276, error in (no error)=w279) -> (notifier out=w277:refnum<notifier>, error out=w278:errorcluster)
          }
        }
      }
      frame #1 {
      }
    }
    n103 = local read "Button States"() -> (w198:T12)
    n104 = Unbundle By Name(w198) -> ("Exit Requested"=w196:bool)
    n105 = Or(x=w196, y=w202) -> (x .or. y?=w197:bool)
  }
  n106 = while {
    shift-right: [w308] -> _
    shift-left: w18 -> [w293]
    shift-right: [w289] -> _
    shift-left: w31 -> [w307]
    tunnel: w45 -> [w304]
    shift-right: [w301] -> _
    shift-left: w15 -> [w302]
    tunnel: w14 -> [w300]
    tunnel: [w297] -> w44
    shift-right: [w294] -> _
    shift-left: w11 -> [w286]
    tunnel: w9 -> [w292]
    stop <- w297 stop-if-true
    # "Gui Events"
    n107 = local read "Button States"() -> (w305:T12)
    n108 = event shown="[0] Timeout" {
      selector: _ -> [_ _ _ _ _ _ _ _ _ _ _ _ _ _ _ _]
      dyn-events: _ -> [_ _ _ _ _ _ _ _ _ _ _ _ _ _ _ _]
      timeout: 200 -> [_ _ _ _ _ _ _ _ _ _ _ _ _ _ _ _]
      tunnel: [Mixed_Mode_Button_Events."Nop" ("MM Control Events") Mixed_Mode_Button_Events."Nop" ("MM Control Events") Mixed_Mode_Button_Events."Nop" ("MM Control Events") Mixed_Mode_Button_Events."Nop" ("MM Control Events") w379 Mixed_Mode_Button_Events."Propose.Accept" ("MM Control Events") Mixed_Mode_Button_Events."Propose.Decline" ("MM Control Events") Mixed_Mode_Button_Events."Execute.Start" ("MM Control Events") Mixed_Mode_Button_Events."Execute.Stop" ("MM Control Events") w412 Mixed_Mode_Button_Events."InputFile.Load" ("MM Control Events") Mixed_Mode_Button_Events."InputFile.Reset" ("MM Control Events") Mixed_Mode_Button_Events."InputFile.Run" ("MM Control Events") Mixed_Mode_Button_Events."Nop" ("MM Control Events") w457 Mixed_Mode_Button_Events."Nop" ("MM Control Events")] -> w309
      tunnel: w307 -> [w342 w358 w366 w371 w376 w389 w394 w399 w404 w413 w420 w429 w436 w450 w462 w467]
      tunnel: [w341 w358 w366 w371 w376 w389 w394 w399 w404 w413 w419 w428 w436 w449 w462 w466] -> w290
      tunnel: w305 -> [_ _ _ _ _ _ _ _ _ _ w422 _ w435 _ w460 _]
      tunnel: [_ _ _ _ _ _ _ _ _ _ w418 _ w434 _ w454 _] -> w303
      tunnel: [_ _ _ _ _ _ _ _ _ _ _ _ _ _ _ w472] -> w299
      tunnel: w302 -> [w344 w357 w365 w370 w378 w387 w392 w397 w402 w411 w423 w430 w438 w447 w461 w468]
      tunnel: [w340 w357 w365 w370 w378 w387 w392 w397 w402 w411 w423 w430 w438 w448 w461 w469] -> w301
      tunnel: w300 -> [w343 _ _ _ _ _ _ _ _ _ _ _ _ w451 _ w465]
      tunnel: [Mixed_Mode_GUI_Update_Type."Nop" ("MM GUI Update Type") Mixed_Mode_GUI_Update_Type."Nop" ("MM GUI Update Type") Mixed_Mode_GUI_Update_Type."Propose.Auto" ("MM GUI Update Type") Mixed_Mode_GUI_Update_Type."Execute.Auto" ("MM GUI Update Type") w377 Mixed_Mode_GUI_Update_Type."Nop" ("MM GUI Update Type") Mixed_Mode_GUI_Update_Type."Nop" ("MM GUI Update Type") Mixed_Mode_GUI_Update_Type."Nop" ("MM GUI Update Type") Mixed_Mode_GUI_Update_Type."Nop" ("MM GUI Update Type") Mixed_Mode_GUI_Update_Type."Nop" ("MM GUI Update Type") Mixed_Mode_GUI_Update_Type."Input File Loaded" ("MM GUI Update Type") Mixed_Mode_GUI_Update_Type."Nop" ("MM GUI Update Type") Mixed_Mode_GUI_Update_Type."RunInputFile" ("MM GUI Update Type") Mixed_Mode_GUI_Update_Type."Nop" ("MM GUI Update Type") Mixed_Mode_GUI_Update_Type."NTCP Server" ("MM GUI Update Type") Mixed_Mode_GUI_Update_Type."Nop" ("MM GUI Update Type")] -> w291
      tunnel: [_ _ w363 w369 _ _ _ _ _ _ w416 _ w432 _ w453 _] -> w287
      event #0 {
        n109 = event-data() -> ()  [unwired: 1 in, 2 out]
        n110 = local read "Cartesian Type"() -> (w337:bool)
        n111 = call "App Status Globals.vi"("App Status Actions"=App_Status_Actions."Get Status") -> ("App Status Out"=w338:T37)  [unwired: 5 in, 9 out]
        n112 = Unbundle By Name(w338) -> ("Cartesian Type"=w335:bool)
        n113 = Not Equal?(x=w337, y=w335) -> (x != y?=w336:bool)
        n114 = case shown="False" w336 {
          tunnel: w344 -> [w346 w352]
          tunnel: w343 -> [_ w351]
          tunnel: w342 -> [w347 w350]
          tunnel: [w347 w349] -> w341
          tunnel: [w346 w348] -> w340
          frame #0 {
          }
          frame #1 {
            n115 = Bundle By Name(cluster=w351, "Command"=MM_Widget_Parameter_Changes."Cartesian Type Changed") -> (w354:T30)
            n116 = Send Notification(notification=w354, notifier=w352, error in (no error)=w350) -> (notifier out=w348:refnum<notifier>, error out=w349:errorcluster)
          }
        }
      }
      event #1 {
        n117 = event-data() -> ()  [unwired: 1 in, 7 out]
        n118 = local read "Mixed Mode Status"() -> (w361:T7)
        n119 = local read "Target Pattern"() -> (w362:T17)
        n120 = call "Apply Target Pattern.vi"("Mixed Mode Status"=w361, "Target Pattern"=w362) -> ("Targets"=w359:T3[])  [unwired: 9 in]
        n121 = local write "Targets"(w359) -> ()
        n122 = event-data("Discard?"=TRUE) -> ()  [unwired: 1 in, 1 out]
      }
      event #2 {
        n123 = event-data() -> ("NewVal"=w363:bool)  [unwired: 1 in, 4 out]
      }
      event #3 {
        n124 = event-data() -> ("NewVal"=w369:bool)  [unwired: 1 in]
      }
      event #4 {
        n125 = event-data() -> ()  [unwired: 1 in, 7 out]
        n126 = call "Can Switch Control Types.vi"("DAO Actions"=DAO_Actions."Get") -> ("Can Switch Out"=w374:bool)  [unwired: 10 in]
        n127 = case shown="False" w374 {
          tunnel: [Mixed_Mode_Button_Events."Nop" ("MM Control Events") Mixed_Mode_Button_Events."ControlType.Changed" ("MM Control Events")] -> w379
          tunnel: [Mixed_Mode_GUI_Update_Type."Nop" ("MM GUI Update Type") Mixed_Mode_GUI_Update_Type."All Autos Off" ("MM GUI Update Type")] -> w377
          tunnel: [TRUE _] -> w373
          frame #0 {
          }
          frame #1 {
          }
        }
        n128 = event-data("Discard?"=w373) -> ()  [unwired: 4 in, 1 out]
      }
      event #5 {
        n129 = event-data() -> ()  [unwired: 1 in, 7 out]
        n130 = event-data("Discard?"=TRUE) -> ()  [unwired: 1 in, 1 out]
      }
      event #6 {
        n131 = event-data() -> ()  [unwired: 1 in, 7 out]
        n132 = event-data("Discard?"=TRUE) -> ()  [unwired: 1 in, 1 out]
      }
      event #7 {
        n133 = event-data() -> ()  [unwired: 1 in, 7 out]
        n134 = event-data("Discard?"=TRUE) -> ()  [unwired: 1 in, 1 out]
      }
      event #8 {
        n135 = event-data() -> ()  [unwired: 1 in, 7 out]
        n136 = event-data("Discard?"=TRUE) -> ()  [unwired: 1 in, 1 out]
      }
      event #9 {
        n137 = event-data() -> ()  [unwired: 1 in, 2 out]
        n138 = call "Fault List 2 Indicators.vi"("Use LBCB Selector"=FALSE) -> ("Forces"=w406:bool, "Displacement"=w407:bool)  [unwired: 8 in, 1 out]
        n139 = Or(x=w407, y=w406) -> (x .or. y?=w408:bool)
        n140 = case shown="False" w408 {
          tunnel: [Mixed_Mode_Button_Events."Nop" ("MM Control Events") Mixed_Mode_Button_Events."TargetSet" ("MM Control Events")] -> w412
          frame #0 {
          }
          frame #1 {
          }
        }
        n141 = event-data("Discard?"=TRUE) -> ()  [unwired: 1 in, 1 out]
      }
      event #10 {
        w416 = TRUE ("Input File Loaded")
        n142 = event-data() -> ()  [unwired: 1 in, 7 out]
        n143 = call "Input Files.vi"("error in (no error)"=w420) -> ("error out"=w419:errorcluster)  [unwired: 10 in]
        n144 = Bundle By Name(cluster=w422, "Input File Loaded"=w416) -> (w418:T12)
        n145 = event-data("Discard?"=TRUE) -> ()  [unwired: 1 in, 1 out]
      }
      event #11 {
        n146 = event-data() -> ()  [unwired: 1 in, 7 out]
        n147 = call "Input File Step Iterator.vi"("error in (no error)"=w429, "Input File Step Actions"=Input_File_Step_Actions."Reset") -> ("error out"=w428:errorcluster)  [unwired: 4 in, 3 out]
        n148 = event-data("Discard?"=TRUE) -> ()  [unwired: 1 in, 1 out]
      }
      event #12 {
        w432 = TRUE ("Input File Running")
        n149 = event-data() -> ()  [unwired: 1 in, 7 out]
        n150 = Bundle By Name(cluster=w435, "Input File Running"=w432) -> (w434:T12)
        n151 = event-data("Discard?"=TRUE) -> ()  [unwired: 1 in, 1 out]
      }
      event #13 {
        # "GUI is updated\nin the Application\nEvents loop"
        n152 = event-data() -> ()  [unwired: 1 in, 2 out]
        n153 = local read "Cartesian Type"() -> (w441:bool)
        n154 = Bundle By Name(cluster=w451, "Command"=MM_Widget_Parameter_Changes."Cartesian Type Changed") -> (w446:T30)
        n155 = Not(x=w441) -> (.not. x?=w442:bool)
        n156 = call "App Status Globals.vi"("App Status Actions"=App_Status_Actions."Set Cart Type", "Status\nSetting"=w442) -> ()  [unwired: 4 in, 10 out]
        n157 = event-data("Discard?"=TRUE) -> ()  [unwired: 1 in, 1 out]
        n158 = Send Notification(notification=w446, notifier=w447, error in (no error)=w450) -> (notifier out=w448:refnum<notifier>, error out=w449:errorcluster)
      }
      event #14 {
        n159 = event-data() -> ()  [unwired: 1 in, 1 out]
        n160 = local read "Connect Server"() -> (w459:bool)
        n161 = Not(x=w459) -> (.not. x?=w453:bool)
        n162 = Bundle By Name(cluster=w460, "NTCP Server  On"=w453) -> (w454:T12)
        n163 = Select(t=Mixed_Mode_Button_Events."NCTP.ConnectToServer" ("MM Control Events"), s=w453, f=Mixed_Mode_Button_Events."NTCP.DisconnectFromServer") -> (s? t:f=w457:T33)
        n164 = event-data("Discard?"=TRUE) -> ()  [unwired: 1 in, 1 out]
      }
      event #15 {
        # "GUI is updated\nin the Application\nEvents loop"
        n165 = event-data() -> ("NewVal"=w472:bool)  [unwired: 1 in]
        n166 = Bundle By Name(cluster=w465, "Command"=MM_Widget_Parameter_Changes."Stop All") -> (w471:T30)
        n167 = Send Notification(notification=w471, notifier=w468, error in (no error)=w467) -> (notifier out=w469:refnum<notifier>, error out=w466:errorcluster)
      }
    }
    n168 = local read "Button States"() -> (w298:T12)
    n169 = Unbundle By Name(w298) -> ("Exit Requested"=w296:bool)
    n170 = Or(x=w296, y=w299) -> (x .or. y?=w297:bool)
    n171 = case shown="\"Nop\"" w291 {
      selector: w291 -> [_ w316 _]
      tunnel: w286 -> [w311 w319 w323]
      tunnel: [w311 w318 w321] -> w294
      tunnel: w292 -> [_ w317 _]
      tunnel: w290 -> [w310 w314 w322]
      tunnel: [w310 w313 w320] -> w288
      tunnel: w287 -> [_ w312 _]
      frame #0 {
      }
      frame #1 {
        n172 = Bundle By Name(cluster=w317, "MM GUI Update Type"=w316, "State"=w312) -> (w315:T28)
        n173 = Enqueue Element(queue=w319, element=w315, error in (no error)=w314) -> (queue out=w318:refnum<queue>, error out=w313:errorcluster)  [unwired: 1 in, 1 out]
      }
      frame #2 {
        n174 = call "Autos Off.vi"("error in"=w322, "queue in"=w323) -> ("error out"=w320:errorcluster, "queue out"=w321:refnum<queue>)  [unwired: 2 in]
      }
    }
    n175 = case shown="\"Propose.Accept\", Default" w309 {
      selector: w309 -> [w325 _]
      tunnel: w293 -> [w331 w333]
      tunnel: [w330 w333] -> w308
      tunnel: w290 -> [w329 w332]
      tunnel: [w328 w332] -> w306
      tunnel: w304 -> [w327 _]
      tunnel: w303 -> [w324 _]
      frame #0 {
        n176 = Bundle By Name(cluster=w327, "MM Control Events"=w325, "Button States"=w324) -> (w326:T32)
        n177 = Send Notification(notification=w326, notifier=w331, error in (no error)=w329) -> (notifier out=w330:refnum<notifier>, error out=w328:errorcluster)
      }
      frame #1 {
      }
    }
    n178 = call <vilib>:"Merge Errors.vi"("error in 3 (no error)"=w306, "error in 2 (no error)"=w288) -> ("error out"=w289:errorcluster)  [unwired: 5 in]
  }
  n179 = Obtain Notifier(name (unnamed)="Mixed Mode Statuses", notification data type=T7 {"LBCB Target"=[], "MixedModeStates"=enum."Init", "LBCB Convergence"=[], "LBCB Measurements"=[]} ("Mixed Mode Status"), error in (no error)=w31) -> (notifier out=w36:refnum<notifier>, error out=w35:errorcluster)  [unwired: 1 in, 1 out]
  n180 = Obtain Queue(name (unnamed)="Mixed Mode State", element data type=w4, error in (no error)=w31) -> (queue out=w32:refnum<queue>, error out=w21:errorcluster)  [unwired: 2 in, 1 out]
  n181 = Obtain Queue(name (unnamed)="MCL States", element data type=MCL_States."MCL Idle" ("MCL States"), error in (no error)=w21) -> (queue out=w17:refnum<queue>, error out=w3:errorcluster)  [unwired: 2 in, 1 out]
  n182 = Obtain Queue(name (unnamed)="Proxy Mixed Mode State", element data type=w4, error in (no error)=w3) -> (queue out=w1:refnum<queue>, error out=w2:errorcluster)  [unwired: 2 in, 1 out]
  n183 = while {
    tunnel: [w492] -> w23
    shift-right: [w490] -> _
    shift-left: Input_File_States."InputFile.Idle" ("Input File States") -> [w491]
    shift-right: [w481] -> _
    shift-left: w18 -> [w482]
    shift-right: [w486] -> _
    shift-left: w20 -> [w487]
    shift-right: [w485] -> _
    shift-left: w11 -> [w488]
    shift-right: [w477] -> _
    shift-left: w17 -> [w478]
    shift-right: [w479] -> _
    shift-left: w13 -> [w480]
    tunnel: w9 -> [w483]
    stop <- w492 stop-if-true
    n184 = local read "Mixed Mode Control Tabs"() -> (w476:enum32{"Manual", "Input File", "NTCP"})
    n185 = local read "Button States"() -> (w493:T12)
    n186 = Unbundle By Name(w493) -> ("Auto-Accept Enabled"=w475:bool, "Auto-Start Enabled"=w474:bool, "Input File Loaded"=w489:bool, "Exit Requested"=w492:bool)
    n187 = case shown="\"Manual\", Default" w476 {
      tunnel: w491 -> [_ w517]
      tunnel: [Input_File_States."InputFile.Idle" ("Input File States") w516] -> w490
      tunnel: w489 -> [_ w515]
      tunnel: w488 -> [w497 w514]
      tunnel: w487 -> [w496 w513]
      tunnel: [w496 w512] -> w486
      tunnel: [w497 w511] -> w485
      tunnel: 200 ("timeout in ms (-1)") -> [_ w503]
      tunnel: w483 -> [_ w510]
      tunnel: w482 -> [w498 w509]
      tunnel: [w498 w508] -> w481
      tunnel: w480 -> [w494 w507]
      tunnel: [w494 w506] -> w479
      tunnel: w478 -> [w495 w505]
      tunnel: [w495 w504] -> w477
      tunnel: w475 -> [_ w502]
      tunnel: w474 -> [_ w501]
      frame #0 {
        n188 = Wait Until Next ms Multiple(millisecond multiple=u32 200) -> ()  [unwired: 1 out]
      }
      frame #1 {
        n189 = case shown="\"InputFile.WaitForMclDone\"" w517 {
          selector: w517 -> [w526 w529 _ _ w617 w637 w661 w687 _]
          tunnel: [w528 w530 w584 w604 w618 w638 w668 w689 Input_File_States."InputFile.Idle" ("Input File States")] -> w516
          tunnel: w515 -> [w527 _ _ _ _ _ _ _ _]
          tunnel: w514 -> [w523 w536 w583 w612 w624 w643 w670 w691 w707]
          tunnel: w513 -> [w524 w541 w577 w598 w623 w642 w677 w684 w705]
          tunnel: [w524 w531 w576 w593 w622 w633 w667 w683 w697] -> w512
          tunnel: [w523 w532 w583 w591 w621 w640 w670 w691 w698] -> w511
          tunnel: w510 -> [_ w535 _ w589 _ _ _ _ w710]
          tunnel: w509 -> [w520 w542 w580 w606 w625 w644 w675 w685 w704]
          tunnel: [w520 w540 w579 w605 w620 w641 w674 w685 w704] -> w508
          tunnel: w507 -> [w522 w538 w581 w600 w616 w632 w676 w686 w702]
          tunnel: [w522 w538 w581 w600 w616 w631 w673 w686 w702] -> w506
          tunnel: w505 -> [w521 w539 w582 w601 w615 w635 w672 w693 w703]
          tunnel: [w521 w539 w582 w601 w615 w635 w671 w692 w703] -> w504
          tunnel: w503 -> [_ w533 w578 w599 w614 w636 w664 w688 _]
          tunnel: w502 -> [_ _ _ _ w613 _ _ _ _]
          tunnel: w501 -> [_ _ _ _ _ w630 _ _ _]
          frame #0 {
            n190 = call "Can Switch Control Types.vi"("Can Switch In"=TRUE, "DAO Actions"=DAO_Actions."Set") -> ()  [unwired: 9 in, 1 out]
            n191 = Select(t=Input_File_States."InputFile.WaitForRunning" ("Input File States"), s=w527, f=w526) -> (s? t:f=w528:T19)
          }
          frame #1 {
            n192 = call "Input File Run or Stop.vi"("timeout"=w533, "error in (no error)"=w541, "MM Button Events In"=w542) -> ("error out"=w534:errorcluster, "Running"=w537:T42, "Button Events Out"=w540:refnum<notifier>)  [unwired: 6 in]
            n193 = case shown="\"Stop\"" w537 {
              tunnel: w536 -> [w545 w550 w562]
              tunnel: w535 -> [_ w555 w567]
              tunnel: w534 -> [w544 w551 w563]
              tunnel: w533 -> [_ w549 w561]
              tunnel: [w545 w548 w560] -> w532
              tunnel: [w544 w547 w559] -> w531
              tunnel: [w543 Input_File_States."InputFile.WaitForRunning" ("Input File States") Input_File_States."InputFile.StepsAvailable" ("Input File States")] -> w530
              tunnel: w529 -> [w543 _ _]
              frame #0 {
              }
              frame #1 {
                n194 = Bundle By Name(cluster=w555, "MM GUI Update Type"=Mixed_Mode_GUI_Update_Type."RunInputFile", "State"=FALSE) -> (w554:T28)
                n195 = Enqueue Element(queue=w550, element=w554, timeout in ms (-1)=w549, error in (no error)=w551) -> (queue out=w548:refnum<queue>, error out=w547:errorcluster)  [unwired: 1 out]
              }
              frame #2 {
                n196 = Bundle By Name(cluster=w567, "MM GUI Update Type"=Mixed_Mode_GUI_Update_Type."RunInputFile", "State"=TRUE) -> (w566:T28)
                n197 = call "Can Switch Control Types.vi"("Can Switch In"=FALSE, "DAO Actions"=DAO_Actions."Set") -> ()  [unwired: 9 in, 1 out]
                n198 = Enqueue Element(queue=w562, element=w566, timeout in ms (-1)=w561, error in (no error)=w563) -> (queue out=w560:refnum<queue>, error out=w559:errorcluster)  [unwired: 1 out]
              }
            }
          }
          frame #2 {
            w571 = Input_File_States."InputFile.StopRunning" ("t")
            n199 = call "Input File Run or Stop.vi"("timeout"=w578, "error in (no error)"=w577, "MM Button Events In"=w580) -> ("error out"=w576:errorcluster, "Running"=w569:T42, "Button Events Out"=w579:refnum<notifier>)  [unwired: 6 in]
            n200 = Not Equal?(x=w569, y=Run_Or_Stop_Result."Stop") -> (x != y?=w570:bool)
            n201 = call "Input File Step Iterator.vi"("Input File Step Actions"=Input_File_Step_Actions."Next Step") -> ("End of Input File"=w574:bool)  [unwired: 5 in, 3 out]
            n202 = Select(t=w571, s=w574, f=Input_File_States."InputFile.LoadStep") -> (s? t:f=w573:T19)
            n203 = Select(t=w573, s=w570, f=w571) -> (s? t:f=w584:T19)
          }
          frame #3 {
            n204 = call "Input File Step Iterator.vi"("Input File Step Actions"=Input_File_Step_Actions."Get Step") -> ("Last Step"=w587:i32, "Next Step"=w609:T43)  [unwired: 5 in, 2 out]
            n205 = Unbundle By Name(w609) -> ("Targets"=w608:T3[], "Step Number"=w588:u32)
            n206 = call "Input File Run or Stop.vi"("timeout"=w599, "error in (no error)"=w598, "MM Button Events In"=w606) -> ("Running"=w596:T42, "Button Events Out"=w605:refnum<notifier>)  [unwired: 6 in, 1 out]
            n207 = Bundle By Name(cluster=w589, "MM GUI Update Type"=Mixed_Mode_GUI_Update_Type."Targets", "Targets"=w608) -> (w607:T28)
            n208 = Format Into String(format string="%d out of %d", w588, w587) -> (resulting string=w585:string)  [unwired: 2 in, 1 out]
            n209 = Bundle By Name(cluster=w589, "MM GUI Update Type"=Mixed_Mode_GUI_Update_Type."TestStats", "Step"=w585) -> (w590:T28)
            n210 = Enqueue Element(queue=w612, element=w607, timeout in ms (-1)=w599, error in (no error)=w598) -> (queue out=w592:refnum<queue>, error out=w593:errorcluster)  [unwired: 1 out]
            n211 = Equal?(x=w596, y=Run_Or_Stop_Result."Stop") -> (x = y?=w595:bool)
            n212 = Enqueue Element(queue=w592, element=w590, error in (no error)=w593) -> (queue out=w591:refnum<queue>)  [unwired: 1 in, 2 out]
            n213 = Select(t=Input_File_States."InputFile.StopRunning" ("f"), s=w595, f=Input_File_States."InputFile.WaitForAccept") -> (s? t:f=w604:T19)
          }
          frame #4 {
            n214 = call "Accept Or Decline.vi"("timeout"=w614, "error in (no error)"=w623, "AutoAccept"=w613, "MM Gui Updates In"=w624, "MM Button Events In"=w625) -> ("error out"=w622:errorcluster, "Accepted or Declined"=w619:T44, "MM Gui Updates Out"=w621:refnum<queue>, "Button Events Out"=w620:refnum<notifier>)  [unwired: 3 in]
            n215 = case shown="\"Accepted\"" w619 {
              tunnel: [w626 Input_File_States."InputFile.WaitForStart" ("f") Input_File_States."InputFile.StopRunning" ("f") Input_File_States."InputFile.StopRunning" ("f")] -> w618
              tunnel: w617 -> [w626 _ _ _]
              frame #0 {
              }
              frame #1 {
              }
              frame #2 {
              }
              frame #3 {
              }
            }
          }
          frame #5 {
            n216 = call "Start Or Stop.vi"("timeout"=w636, "error in (no error)"=w642, "AutoStart"=w630, "MM Gui Updates In"=w643, "MM Button Events In"=w644) -> ("error out"=w634:errorcluster, "Start or Stop"=w639:T44, "MM Gui Updates Out"=w640:refnum<queue>, "Button Events Out"=w641:refnum<notifier>)  [unwired: 3 in]
            n217 = case shown="\"Accepted\"" w639 {
              tunnel: [w647 Input_File_States."InputFile.WaitForMclRamp" ("f") Input_File_States."InputFile.StopRunning" ("f") Input_File_States."InputFile.StopRunning" ("f")] -> w638
              tunnel: w637 -> [w647 _ _ _]
              tunnel: w634 -> [w645 w653 w655 w658]
              tunnel: [w645 w652 w655 w658] -> w633
              tunnel: w632 -> [w646 w651 w656 w659]
              tunnel: [w646 w650 w656 w659] -> w631
              frame #0 {
              }
              frame #1 {
                n218 = local read "Targets"() -> (w648:T3[])
                n219 = local read "Ramp Times"() -> (w649:cluster{"Displacement":T15, "Force":T15})
                n220 = call "Send Mixed Mode Command.vi"("Targets"=w648, "MCL Command In"=w651, "Ramp Times"=w649, "error in"=w653) -> ("MCL Command Out"=w650:refnum<queue>, "error out"=w652:errorcluster)  [unwired: 1 in]
              }
              frame #2 {
              }
              frame #3 {
              }
            }
          }
          frame #6 {
            n221 = call "Monitor for Stop.vi"("timeout"=w664, "error in (no error)"=w677, "Mixed Mode Commands In"=w676, "MM Button Events In"=w675) -> ("error out"=w665:errorcluster, "Mixed Mode Commands Out"=w673:refnum<queue>, "Stop Requests"=w663:T45, "Button Events Out"=w674:refnum<notifier>)  [unwired: 4 in]
            n222 = case shown="\"Stop Requested\", Default" w663 {
              tunnel: [w678 Input_File_States."InputFile.StopRunning" ("f")] -> w662
              tunnel: w661 -> [w678 _]
              frame #0 {
              }
              frame #1 {
              }
            }
            n223 = call "Done Or Abort.vi"("timeout"=w664, "MCL State In"=w672) -> ("error out"=w666:errorcluster, "MCL State"=w669:T46, "MCL State Out"=w671:refnum<queue>)  [unwired: 2 in]
            n224 = case shown="\"Abort\"" w669 {
              tunnel: [Input_File_States."InputFile.StepsAvailable" ("f") Input_File_States."InputFile.StopRunning" ("f") w682] -> w668
              tunnel: w662 -> [_ _ w682]
              frame #0 {
              }
              frame #1 {
              }
              frame #2 {
              }
            }
            n225 = call <vilib>:"Merge Errors.vi"("error in 3 (no error)"=w666, "error in 1 (no error)"=w665) -> ("error out"=w667:errorcluster)  [unwired: 5 in]
          }
          frame #7 {
            n226 = call "MCL Ramping.vi"("error in (no error)"=w684, "timeout"=w688, "MCL State In"=w693) -> ("error out"=w683:errorcluster, "Is Ramping?"=w690:bool, "MCL State Out"=w692:refnum<queue>)  [unwired: 1 in]
            n227 = case shown="True" w690 {
              tunnel: [w694 Input_File_States."InputFile.WaitForMclDone" ("Input File States")] -> w689
              tunnel: w687 -> [w694 _]
              frame #0 {
              }
              frame #1 {
              }
            }
          }
          frame #8 {
            n228 = Bundle By Name(cluster=w710, "MM GUI Update Type"=Mixed_Mode_GUI_Update_Type."RunInputFile", "State"=FALSE) -> (w706:T28)
            n229 = call "Input File Step Iterator.vi"("Input File Step Actions"=Input_File_Step_Actions."Backup") -> ()  [unwired: 5 in, 4 out]
            n230 = Enqueue Element(queue=w707, element=w706, error in (no error)=w705) -> (queue out=w700:refnum<queue>, error out=w699:errorcluster)  [unwired: 1 in, 1 out]
            n231 = call "Autos Off.vi"("error in"=w699, "queue in"=w700) -> ("error out"=w697:errorcluster, "queue out"=w698:refnum<queue>)  [unwired: 2 in]
          }
        }
      }
    }
    "Input File States" <- w490
  }
  n232 = while {
    shift-right: [w723] -> _
    shift-left: w18 -> [w725]
    shift-right: [w721] -> _
    shift-left: w21 -> [w724]
    shift-right: [w720] -> _
    shift-left: w11 -> [w722]
    shift-right: [w717] -> _
    shift-left: w17 -> [w719]
    shift-right: [w713] -> _
    shift-left: Manual_States."Manual.Idle" ("Manual States") -> [w726]
    shift-right: [w715] -> _
    shift-left: w13 -> [w716]
    tunnel: [w714] -> w24
    stop <- w714 stop-if-true
    # "Manual States"
    n233 = local read "Mixed Mode Control Tabs"() -> (w712:enum32{"Manual", "Input File", "NTCP"})
    n234 = local read "Button States"() -> (w727:T12)
    n235 = Unbundle By Name(w727) -> ("Auto-Start Enabled"=w711:bool, "Exit Requested"=w714:bool)
    n236 = case shown="\"Input File\", Default" w712 {
      tunnel: [w738 Manual_States."Manual.Idle" ("Manual States")] -> w713
      tunnel: w726 -> [w741 _]
      tunnel: w725 -> [w740 w848]
      tunnel: w724 -> [w739 w847]
      tunnel: [w737 w848] -> w723
      tunnel: w722 -> [w736 w846]
      tunnel: [w735 w847] -> w721
      tunnel: [w734 w846] -> w720
      tunnel: w719 -> [w733 w845]
      tunnel: 200 ("timeout in ms (-1)") -> [w732 _]
      tunnel: [w731 w845] -> w717
      tunnel: w716 -> [w730 w844]
      tunnel: [w729 w844] -> w715
      tunnel: w711 -> [w728 _]
      frame #0 {
        n237 = case shown="\"Manual.WaitForMclDone\"" w741 {
          selector: w741 -> [_ _ _ w808 w828 _]
          tunnel: w740 -> [w754 w776 w799 w810 w823 w843]
          tunnel: w739 -> [w753 w774 w797 w811 w824 w838]
          tunnel: [w751 w770 Manual_States."Manual.WaitForMclDone" ("Manual States") w814 w829 Manual_States."Manual.Idle" ("Manual States")] -> w738
          tunnel: [w750 w773 w799 w809 w823 w843] -> w737
          tunnel: w736 -> [w746 w775 w798 w816 w831 w839]
          tunnel: [w747 w766 w801 w806 w826 w836] -> w735
          tunnel: [w746 w772 w798 w816 w831 w837] -> w734
          tunnel: w733 -> [w745 w769 w803 w819 w833 w842]
          tunnel: w732 -> [w748 w764 _ w807 w827 _]
          tunnel: [w745 w769 w803 w818 w832 w842] -> w731
          tunnel: w730 -> [w744 w768 w802 w813 w825 w840]
          tunnel: [w744 w765 w800 w812 w825 w840] -> w729
          tunnel: w728 -> [_ w763 _ _ _ _]
          frame #0 {
            n238 = call "Can Switch Control Types.vi"("Can Switch In"=TRUE, "DAO Actions"=DAO_Actions."Set") -> ()  [unwired: 9 in, 1 out]
            n239 = Wait on Notification(notifier=w754, timeout in ms (-1)=w748, error in (no error)=w753) -> (notifier out=w750:refnum<notifier>, notification=w749:T32, timed out?=w752:bool, error out=w747:errorcluster)  [unwired: 1 in]
            n240 = case shown="False" w752 {
              tunnel: [w755 Manual_States."Manual.Idle" ("Manual States")] -> w751
              tunnel: w749 -> [w757 _]
              frame #0 {
                n241 = Unbundle By Name(w757) -> ("MM Control Events"=w756:T33)
                n242 = case shown="\"Control.Enabled\"" w756 {
                  tunnel: [Manual_States."Manual.WaitForStart" ("t") Manual_States."Manual.Idle" ("Manual States") Manual_States."Manual.InitialPosition" ("t") Manual_States."Manual.InitialPosition" ("t")] -> w755
                  frame #0 {
                  }
                  frame #1 {
                  }
                  frame #2 {
                  }
                  frame #3 {
                  }
                }
              }
              frame #1 {
              }
            }
          }
          frame #1 {
            n243 = call "Start Or Stop.vi"("timeout"=w764, "error in (no error)"=w774, "AutoStart"=w763, "MM Gui Updates In"=w775, "MM Button Events In"=w776) -> ("error out"=w767:errorcluster, "Start or Stop"=w771:T44, "MM Gui Updates Out"=w772:refnum<queue>, "Button Events Out"=w773:refnum<notifier>)  [unwired: 3 in]
            n244 = case shown="\"Accepted\"" w771 {
              tunnel: [Manual_States."Manual.WaitForStart" ("Manual States") Manual_States."Manual.WaitForMclRamp" ("Manual States") Manual_States."Manual.Abort" ("Manual States") Manual_States."Manual.Abort" ("Manual States")] -> w770
              tunnel: w768 -> [w777 w787 w790 w793]
              tunnel: w767 -> [w778 w785 w789 w792]
              tunnel: [w778 w784 w789 w792] -> w766
              tunnel: [w777 w783 w790 w793] -> w765
              frame #0 {
              }
              frame #1 {
                n245 = local read "Ramp Times"() -> (w786:cluster{"Displacement":T15, "Force":T15})
                n246 = local read "Targets"() -> (w782:T3[])
                n247 = call "Send Mixed Mode Command.vi"("Targets"=w782, "MCL Command In"=w787, "Ramp Times"=w786, "error in"=w785) -> ("MCL Command Out"=w783:refnum<queue>, "error out"=w784:errorcluster)  [unwired: 1 in]
                n248 = call "Can Switch Control Types.vi"("Can Switch In"=FALSE, "DAO Actions"=DAO_Actions."Set") -> ()  [unwired: 9 in, 1 out]
              }
              frame #2 {
              }
              frame #3 {
              }
            }
          }
          frame #2 {
            n249 = call "Can Switch Control Types.vi"("Can Switch In"=FALSE, "DAO Actions"=DAO_Actions."Set") -> ()  [unwired: 9 in, 1 out]
            n250 = call "Send Initial Position Command.vi"("MCL Command In"=w802, "error in"=w797) -> ("MCL Command Out"=w800:refnum<queue>, "error out"=w801:errorcluster)  [unwired: 3 in]
          }
          frame #3 {
            n251 = call "Done Or Abort.vi"("timeout"=w807, "MCL State In"=w819) -> ("error out"=w817:errorcluster, "MCL State"=w815:T46, "MCL State Out"=w818:refnum<queue>)  [unwired: 2 in]
            n252 = call "Monitor for Stop.vi"("timeout"=w807, "error in (no error)"=w811, "Mixed Mode Commands In"=w813, "MM Button Events In"=w810) -> ("error out"=w805:errorcluster, "Mixed Mode Commands Out"=w812:refnum<queue>, "Button Events Out"=w809:refnum<notifier>)  [unwired: 4 in, 1 out]
            n253 = case shown="\"Still Running\"" w815 {
              tunnel: [Manual_States."Manual.Idle" ("Manual States") Manual_States."Manual.Abort" ("Manual States") w822] -> w814
              tunnel: w808 -> [_ _ w822]
              frame #0 {
              }
              frame #1 {
              }
              frame #2 {
              }
            }
            n254 = call <vilib>:"Merge Errors.vi"("error in 3 (no error)"=w817, "error in 1 (no error)"=w805) -> ("error out"=w806:errorcluster)  [unwired: 5 in]
          }
          frame #4 {
            n255 = call "MCL Ramping.vi"("error in (no error)"=w824, "timeout"=w827, "MCL State In"=w833) -> ("error out"=w826:errorcluster, "Is Ramping?"=w830:bool, "MCL State Out"=w832:refnum<queue>)  [unwired: 1 in]
            n256 = case shown="True" w830 {
              tunnel: [w834 Manual_States."Manual.WaitForMclDone" ("Manual States")] -> w829
              tunnel: w828 -> [w834 _]
              frame #0 {
              }
              frame #1 {
              }
            }
          }
          frame #5 {
            n257 = call "Autos Off.vi"("error in"=w838, "queue in"=w839) -> ("error out"=w836:errorcluster, "queue out"=w837:refnum<queue>)  [unwired: 2 in]
          }
        }
      }
      frame #1 {
        n258 = Wait Until Next ms Multiple(millisecond multiple=u32 200) -> ()  [unwired: 1 out]
      }
    }
    n259 = local write "Manual States"(w713) -> ()
  }
  n260 = call "Names Data Set.vi"("Name Actions"=Name_Actions."Get Names") -> ("External Sensor Names"=w33:string[])  [unwired: 1 in, 13 out]
  n261 = while {
    shift-right: [w860] -> _
    shift-left: w36 -> [w863]
    shift-right: [w859] -> _
    shift-left: w35 -> [w862]
    tunnel: w33 -> [w856]
    tunnel: [w855] -> w28
    stop <- w855 stop-if-true
    # "Gui Continuous\nUpdates"
    n262 = local read "Channel Data Tables"() -> (w864:T16)
    n263 = Wait on Notification(notifier=w863, timeout in ms (-1)=200, error in (no error)=w862) -> (notifier out=w860:refnum<notifier>, notification=w857:T7, timed out?=w858:bool, error out=w859:errorcluster)  [unwired: 1 in]
    n264 = case shown="False" w858 {
      tunnel: w864 -> [w876 _]
      tunnel: w857 -> [w872 _]
      tunnel: w856 -> [w874 _]
      frame #0 {
        n265 = Unbundle By Name(w872) -> ("LBCB Measurements"=w873:T11[])
        n266 = local read "Cartesian Type"() -> (w870:bool)
        n267 = case shown="\"Cartesian\"" w876 {
          tunnel: w874 -> [_ w883 _]
          tunnel: w870 -> [w877 w882 _]
          frame #0 {
            n268 = call "Generate Data Tables.vi"("LBCB Number"=LBCB_Number."LBCB2", "Cartesian Type"=w877) -> ("Cartesian Table"=w879:dbl[][])  [unwired: 1 in, 3 out]
            n269 = call "Generate Data Tables.vi"("LBCB Number"=LBCB_Number."LBCB1", "Cartesian Type"=w877) -> ("Cartesian Table"=w878:dbl[][])  [unwired: 1 in, 3 out]
            n270 = local write "LBCB 2 Cartesian Space"(w879) -> ()
            n271 = local write "LBCB 1 Cartesian Space"(w878) -> ()
          }
          frame #1 {
            n272 = call "Generate External Sensors Table.vi"("External Sensor Names"=w883, "WithOffset"=w882) -> ("External Sensors"=w884:cluster{"Name":string, "Value":dbl}[])  [unwired: 1 in, 8 out]
            n273 = local write "External Sensors"(w884) -> ()
          }
          frame #2 {
            w889 = FALSE ("Cartesian Type")
            # "Cartesian Type ignored\nbecause we are  using \nActuator Space"
            n274 = call "Generate Data Tables.vi"("LBCB Number"=LBCB_Number."LBCB2", "Cartesian Type"=w889) -> ("Actuator Table"=w885:dbl[][])  [unwired: 1 in, 3 out]
            n275 = call "Generate Data Tables.vi"("LBCB Number"=LBCB_Number."LBCB1", "Cartesian Type"=w889) -> ("Actuator Table"=w886:dbl[][])  [unwired: 1 in, 3 out]
            n276 = local write "LBCB 1 Actuator Space"(w886) -> ()
            n277 = local write "LBCB 2 Actuator Space"(w885) -> ()
          }
        }
        n278 = local read "Targets"() -> (w875:T3[])
        n279 = call "Measurements 2 Target Arrays.vi"("LBCB Command Data"=w873, "Target  Inputs"=w875) -> ("Target  Outputs"=w867:T3[])  [unwired: 9 in]
        n280 = local write "Mixed Mode Status"(w872) -> ()
        n281 = Select(t=enum16{" +", " - "}." - " ("Direction"), s=w870, f=enum16{" +", " - "}." +") -> (s? t:f=w871:enum16{" +", " - "})
        n282 = call "Local2Global Target Values.vi"("Direction"=w871, "Target  Inputs"=w867) -> ("Target  Outputs"=w866:T3[])  [unwired: 9 in]
        n283 = local write "Current Values"(w866) -> ()
      }
      frame #1 {
      }
    }
    n284 = call "App Status Globals.vi"("App Status Actions"=App_Status_Actions."Get Status") -> ("App Status Out"=w853:T37)  [unwired: 13 in, 1 out]
    n285 = Unbundle By Name(w853) -> ("NTCP Link"=w852:bool)
    n286 = local write "Connected"(w852) -> ()
    n287 = call "Messages.vi"() -> ("Messages"=w851:string)  [unwired: 1 in, 10 out]
    n288 = local write "Messages"(w851) -> ()
    n289 = local read "Button States"() -> (w865:T12)
    n290 = Unbundle By Name(w865) -> ("Exit Requested"=w855:bool)
  }
  n291 = while {
    shift-right: [w905] -> _
    shift-left: _ -> [w908]
    shift-right: [w906] -> _
    shift-left: _ -> [w907]
    shift-right: [w903] -> _
    shift-left: w8 -> [w904]
    shift-right: [w912] -> _
    shift-left: w18 -> [w916]
    shift-right: [w911] -> _
    shift-left: w11 -> [w915]
    shift-right: [w910] -> _
    shift-left: w17 -> [w914]
    shift-right: [w909] -> _
    shift-left: w13 -> [w913]
    tunnel: w9 -> [w901]
    shift-right: [w900] -> _
    shift-left: NTCP_Mixed_Mode_States."Ntcp.Off" ("NTCP MM States") -> [w918]
    tunnel: T23 {"NTCP commands"=enum."propose", "Transaction ID"="", "Control Point"="", "Accepted"=FALSE} ("NTCP Message") -> [w899]
    tunnel: [w898] -> w16
    shift-right: [w896] -> _
    shift-left: w15 -> [w897]
    tunnel: w14 -> [w895]
    shift-right: [w890] -> _
    shift-left: FALSE -> [w891]
    stop <- w898 stop-if-true
    # "NTCP States"
    n292 = local read "Button States"() -> (w917:T12)
    n293 = local read "Mixed Mode Control Tabs"() -> (w894:enum32{"Manual", "Input File", "NTCP"})
    n294 = Unbundle By Name(w917) -> ("Auto-Start Enabled"=w893:bool, "Auto-Accept Enabled"=w892:bool, "Exit Requested"=w898:bool)
    n295 = case shown="\"NTCP\"" w894 {
      tunnel: w918 -> [w921 w955]
      tunnel: [w929 w952] -> w912
      tunnel: w916 -> [w929 w953]
      tunnel: [w928 w948] -> w911
      tunnel: w915 -> [w928 w949]
      tunnel: [w927 w945] -> w910
      tunnel: w914 -> [w927 w946]
      tunnel: [w926 w943] -> w909
      tunnel: w913 -> [w926 w944]
      tunnel: [w925 w941] -> w905
      tunnel: w908 -> [w925 w942]
      tunnel: [w924 w939] -> w906
      tunnel: w907 -> [w924 w940]
      tunnel: [w923 w950] -> w903
      tunnel: w904 -> [w923 w951]
      tunnel: 200 ("timeout in ms (-1)") -> [_ w954]
      tunnel: w901 -> [_ w947]
      tunnel: [w921 w938] -> w900
      tunnel: w899 -> [_ w937]
      tunnel: w897 -> [w920 w936]
      tunnel: [w920 w935] -> w896
      tunnel: w895 -> [_ w934]
      tunnel: w893 -> [_ w933]
      tunnel: w892 -> [_ w932]
      tunnel: w891 -> [w919 w931]
      tunnel: [w919 w930] -> w890
      frame #0 {
        n296 = Wait Until Next ms Multiple(millisecond multiple=u32 200) -> ()  [unwired: 1 out]
      }
      frame #1 {
        n297 = case shown="\"Ntcp.WaitForMclRamp\"" w955 {
          selector: w955 -> [w966 _ w1128 w1170 w1212 _ _ _]
          tunnel: w954 -> [w980 w1063 w1120 w1185 w1201 w1266 w1293 _]
          tunnel: w953 -> [w979 w1064 w1138 w1184 w1221 w1276 w1303 w1324]
          tunnel: [w978 w1057 w1136 w1176 w1219 w1273 w1300 w1324] -> w952
          tunnel: w951 -> [w977 w1062 w1134 w1180 w1204 w1268 w1295 w1318]
          tunnel: [w975 w1056 w1122 w1179 w1203 w1256 w1281 w1309] -> w950
          tunnel: w949 -> [w974 w1071 w1137 w1175 w1220 w1270 w1297 w1330]
          tunnel: [w972 w1068 w1135 w1175 w1218 w1270 w1297 w1311] -> w948
          tunnel: w947 -> [w971 w1072 _ _ _ _ _ w1329]
          tunnel: [w970 w1065 w1127 w1174 w1208 w1271 w1298 w1323] -> w945
          tunnel: w946 -> [w970 w1065 w1127 w1174 w1208 w1272 w1299 w1323]
          tunnel: [w969 w1066 w1126 w1173 w1216 w1274 w1301 w1322] -> w943
          tunnel: w944 -> [w969 w1066 w1126 w1173 w1214 w1275 w1302 w1322]
          tunnel: [w962 w1067 w1129 w1172 w1209 w1260 w1287 w1321] -> w941
          tunnel: w942 -> [w959 w1067 w1131 w1172 w1211 w1261 w1286 w1321]
          tunnel: w940 -> [w958 w1078 w1125 w1186 w1205 w1265 w1292 w1320]
          tunnel: [w961 w1076 w1124 w1181 w1206 w1264 w1291 w1320] -> w939
          tunnel: [w967 w1061 w1119 w1169 w1200 w1262 w1282 NTCP_Mixed_Mode_States."Ntcp.Off" ("NTCP MM States")] -> w938
          tunnel: w937 -> [w960 _ w1133 _ w1210 _ _ _]
          tunnel: w936 -> [w964 w1053 w1114 w1166 w1196 w1258 w1290 w1319]
          tunnel: [w963 w1053 w1114 w1166 w1196 w1258 w1290 w1316] -> w935
          tunnel: w934 -> [w965 _ _ _ _ _ _ w1315]
          tunnel: w933 -> [_ _ _ _ w1195 _ _ _]
          tunnel: w932 -> [_ _ w1113 _ _ _ _ _]
          tunnel: w931 -> [w957 w1051 w1112 w1163 w1194 w1257 w1289 w1308]
          tunnel: [w956 w1051 w1112 w1163 w1194 w1257 w1289 w1308] -> w930
          frame #0 {
            n298 = Wait on Notification(notifier=w979, timeout in ms (-1)=w980, error in (no error)=w977) -> (notifier out=w978:refnum<notifier>, notification=w976:T32, timed out?=w968:bool, error out=w973:errorcluster)  [unwired: 1 in]
            n299 = case shown="True" w968 {
              tunnel: w976 -> [w994 _]
              tunnel: [w993 w1025] -> w975
              tunnel: w974 -> [w992 w1027]
              tunnel: w973 -> [w990 w1021]
              tunnel: [w991 w1027] -> w972
              tunnel: w971 -> [w989 _]
              tunnel: [w984 w1028] -> w967
              tunnel: w966 -> [_ w1028]
              tunnel: w965 -> [w987 _]
              tunnel: w964 -> [w986 w1026]
              tunnel: [w985 w1026] -> w963
              tunnel: [w983 w1024] -> w962
              tunnel: [w982 w1023] -> w961
              tunnel: w960 -> [_ w1022]
              tunnel: w959 -> [w983 w1017]
              tunnel: w958 -> [w982 w1018]
              tunnel: w957 -> [w981 w1020]
              tunnel: [w981 w1019] -> w956
              frame #0 {
                n300 = Unbundle By Name(w994) -> ("MM Control Events"=w988:T33)
                n301 = case shown="\"NCTP.ConnectToServer\"" w988 {
                  tunnel: w990 -> [w998 w1002]
                  tunnel: [w998 w1009] -> w993
                  tunnel: w992 -> [w997 w1012]
                  tunnel: [w997 w1011] -> w991
                  tunnel: w989 -> [_ w1010]
                  tunnel: w987 -> [_ w1005]
                  tunnel: w986 -> [w996 w1006]
                  tunnel: [w996 w1000] -> w985
                  tunnel: [NTCP_Mixed_Mode_States."Ntcp.Off" ("NTCP MM States") NTCP_Mixed_Mode_States."Ntcp.WaitForProposal" ("NTCP MM States")] -> w984
                  frame #0 {
                  }
                  frame #1 {
                    n302 = Bundle By Name(cluster=w1005, "Command"=MM_Widget_Parameter_Changes."NTCP Link On") -> (w1003:T30)
                    n303 = Send Notification(notification=w1003, notifier=w1006, error in (no error)=w1002) -> (notifier out=w1000:refnum<notifier>, error out=w1001:errorcluster)
                    n304 = Bundle By Name(cluster=w1010, "MM GUI Update Type"=Mixed_Mode_GUI_Update_Type."NTCP Server", "State"=TRUE) -> (w1007:T28)
                    n305 = call "NoArgumentsLauncher.vi"("error in (no error)"=w1001, "Application"=NoPanelAppTypes."NTCP Socket", "Application Launcher Actions"=Launcher_Actions."Launch") -> ("error out"=w1008:errorcluster)  [unwired: 7 in, 1 out]
                    n306 = Enqueue Element(queue=w1012, element=w1007, error in (no error)=w1008) -> (queue out=w1011:refnum<queue>, error out=w1009:errorcluster)  [unwired: 1 in, 1 out]
                  }
                }
              }
              frame #1 {
                n307 = case shown="False" w1020 {
                  selector: w1020 -> [_ w1048]
                  tunnel: [w1036 w1045] -> w1025
                  tunnel: [w1034 w1046] -> w1024
                  tunnel: [w1033 w1047] -> w1023
                  tunnel: w1022 -> [w1030 _]
                  tunnel: w1021 -> [w1032 w1045]
                  tunnel: [TRUE w1048] -> w1019
                  tunnel: w1018 -> [_ w1047]
                  tunnel: w1017 -> [_ w1046]
                  frame #0 {
                    n308 = call "NTCP Network Parameters DAO.vi"("Persistent DAO Actions"=Persistant_DAO_Actions."Get") -> ("Network Parameters Out"=w1042:T51)  [unwired: 8 in, 2 out]
                    n309 = Unbundle By Name(w1042) -> ("Notification Name"=w1043:string)
                    n310 = Concatenate Strings("To " ("name (unnamed)"), w1043) -> (w1044:string)
                    "To Queue" <- w1044
                    n311 = Concatenate Strings("From " ("name (unnamed)"), w1043) -> (w1040:string)
                    "From Queue" <- w1040
                    n312 = Obtain Queue(name (unnamed)=w1044, element data type=w1030, error in (no error)=w1032) -> (queue out=w1034:refnum<queue>, error out=w1035:errorcluster)  [unwired: 2 in, 1 out]
                    n313 = Obtain Queue(name (unnamed)=w1040, element data type=T1 {"NTCP commands"=enum."propose", "Transaction ID"="", "Control Point"="", "Targets"=[]} ("NTCP Message"), error in (no error)=w1032) -> (queue out=w1033:refnum<queue>, error out=w1037:errorcluster)  [unwired: 2 in, 1 out]
                    n314 = call <vilib>:"Merge Errors.vi"("error in 3 (no error)"=w1037, "error in 2 (no error)"=w1035) -> ("error out"=w1036:errorcluster)  [unwired: 5 in]
                  }
                  frame #1 {
                  }
                }
              }
            }
          }
          frame #1 {
            n315 = Dequeue Element(queue=w1078, timeout in ms (-1)=w1063, error in (no error)=w1062) -> (queue out=w1076:refnum<queue>, element=w1077:T1, timed out?=w1052:bool, error out=w1070:errorcluster)
            "NTCP" <- w1077
            n316 = call "Monitor for NTCP Close.vi"("Skip"=Skip_NTCP_Close_Monitor."Skip NTCP", "timeout"=w1063, "error in (no error)"=w1062, "MM Button Events In"=w1064) -> ("error out"=w1055:errorcluster, "Close Received"=w1059:bool, "Button Events Out"=w1057:refnum<notifier>)  [unwired: 4 in, 1 out]
            n317 = Unbundle By Name(w1077) -> ("NTCP commands"=w1075:T2, "Transaction ID"=w1073:string, "Targets"=w1074:T3[])
            n318 = case shown="False" w1052 {
              tunnel: w1075 -> [w1087 _]
              tunnel: w1074 -> [w1086 _]
              tunnel: w1073 -> [w1085 _]
              tunnel: w1072 -> [w1084 _]
              tunnel: w1071 -> [w1083 w1110]
              tunnel: w1070 -> [w1082 w1109]
              tunnel: [w1081 w1109] -> w1069
              tunnel: [w1080 w1110] -> w1068
              tunnel: [w1079 NTCP_Mixed_Mode_States."Ntcp.WaitForProposal" ("NTCP MM States")] -> w1060
              frame #0 {
                n319 = case shown="\"propose\"" w1087 {
                  tunnel: w1086 -> [w1101 _ _]
                  tunnel: w1085 -> [w1089 _ _]
                  tunnel: w1084 -> [w1097 _ _]
                  tunnel: w1083 -> [w1100 w1105 w1107]
                  tunnel: w1082 -> [w1098 w1104 w1106]
                  tunnel: [w1092 w1104 w1106] -> w1081
                  tunnel: [w1091 w1105 w1107] -> w1080
                  tunnel: [NTCP_Mixed_Mode_States."Ntcp.WaitForAccept" ("NTCP MM States") NTCP_Mixed_Mode_States."Ntcp.WaitForProposal" ("NTCP MM States") NTCP_Mixed_Mode_States."Ntcp.Shutdown" ("NTCP MM States")] -> w1079
                  frame #0 {
                    n320 = Bundle By Name(cluster=w1097, "MM GUI Update Type"=Mixed_Mode_GUI_Update_Type."Targets", "Targets"=w1101) -> (w1099:T28)
                    n321 = Enqueue Element(queue=w1100, element=w1099, error in (no error)=w1098) -> (queue out=w1095:refnum<queue>, error out=w1093:errorcluster)  [unwired: 1 in, 1 out]
                    n322 = call "Extract Step Number from TransID.vi"("TransID"=w1089) -> ("Step"=w1088:string)  [unwired: 10 in]
                    n323 = Bundle By Name(cluster=w1097, "MM GUI Update Type"=Mixed_Mode_GUI_Update_Type."TestStats", "Step"=w1088) -> (w1094:T28)
                    n324 = Enqueue Element(queue=w1095, element=w1094, error in (no error)=w1093) -> (queue out=w1091:refnum<queue>, error out=w1092:errorcluster)  [unwired: 1 in, 1 out]
                  }
                  frame #1 {
                  }
                  frame #2 {
                  }
                }
              }
              frame #1 {
              }
            }
            n325 = call "Can Switch Control Types.vi"("Can Switch In"=TRUE, "DAO Actions"=DAO_Actions."Set") -> ()  [unwired: 9 in, 1 out]
            n326 = call <vilib>:"Merge Errors.vi"("error in 3 (no error)"=w1069, "error in 1 (no error)"=w1055) -> ("error out"=w1056:errorcluster)  [unwired: 5 in]
            n327 = Select(t=NTCP_Mixed_Mode_States."Ntcp.Shutdown", s=w1059, f=w1060) -> (s? t:f=w1061:T20)
          }
          frame #2 {
            n328 = call "Accept Or Decline.vi"("timeout"=w1120, "error in (no error)"=w1134, "AutoAccept"=w1113, "MM Gui Updates In"=w1137, "MM Button Events In"=w1138) -> ("error out"=w1123:errorcluster, "Accepted or Declined"=w1132:T44, "MM Gui Updates Out"=w1135:refnum<queue>, "Button Events Out"=w1136:refnum<notifier>)  [unwired: 3 in]
            n329 = call "Monitor for NTCP Close.vi"("Skip"=Skip_NTCP_Close_Monitor."Skip Button Event", "timeout"=w1120, "error in (no error)"=w1123, "From NTCP In"=w1125) -> ("error out"=w1121:errorcluster, "From NTCP Out"=w1124:refnum<queue>, "Close Received"=w1117:bool)  [unwired: 4 in, 1 out]
            n330 = case shown="\"Abort\"" w1132 {
              tunnel: w1133 -> [_ _ w1153 w1162]
              tunnel: w1131 -> [w1140 w1143 w1150 w1159]
              tunnel: w1123 -> [w1139 w1142 w1148 w1157]
              tunnel: [w1139 w1142 w1147 w1156] -> w1130
              tunnel: [w1140 w1143 w1146 w1155] -> w1129
              tunnel: [w1141 NTCP_Mixed_Mode_States."Ntcp.Shutdown" ("NTCP MM States") NTCP_Mixed_Mode_States."Ntcp.WaitForExecute" ("NTCP MM States") NTCP_Mixed_Mode_States."Ntcp.WaitForProposal" ("NTCP MM States")] -> w1118
              tunnel: w1128 -> [w1141 _ _ _]
              frame #0 {
              }
              frame #1 {
              }
              frame #2 {
                n331 = Bundle By Name(cluster=w1153, "NTCP commands"=NTCP_Commands."propose", "Accepted"=T24 TRUE) -> (w1149:T23)
                n332 = Enqueue Element(queue=w1150, element=w1149, error in (no error)=w1148) -> (queue out=w1146:refnum<queue>, error out=w1147:errorcluster)  [unwired: 1 in, 1 out]
              }
              frame #3 {
                n333 = Bundle By Name(cluster=w1162, "NTCP commands"=NTCP_Commands."propose", "Accepted"=T24 FALSE) -> (w1158:T23)
                n334 = Enqueue Element(queue=w1159, element=w1158, error in (no error)=w1157) -> (queue out=w1155:refnum<queue>, error out=w1156:errorcluster)  [unwired: 1 in, 1 out]
              }
            }
            n335 = Select(t=NTCP_Mixed_Mode_States."Ntcp.Shutdown", s=w1117, f=w1118) -> (s? t:f=w1119:T20)
            n336 = call <vilib>:"Merge Errors.vi"("error in 3 (no error)"=w1121, "error in 2 (no error)"=w1130) -> ("error out"=w1122:errorcluster)  [unwired: 5 in]
          }
          frame #3 {
            n337 = Dequeue Element(queue=w1186, timeout in ms (-1)=w1185, error in (no error)=w1180) -> (queue out=w1181:refnum<queue>, element=w1164:T1, timed out?=w1165:bool, error out=w1177:errorcluster)
            n338 = call "Monitor for NTCP Close.vi"("Skip"=Skip_NTCP_Close_Monitor."Skip NTCP", "timeout"=w1185, "error in (no error)"=w1180, "MM Button Events In"=w1184) -> ("error out"=w1178:errorcluster, "Close Received"=w1168:bool, "Button Events Out"=w1176:refnum<notifier>)  [unwired: 4 in, 1 out]
            n339 = Unbundle By Name(w1164) -> ("NTCP commands"=w1182:T2)
            n340 = local write "NTCP"(w1164) -> ()
            n341 = case shown="False" w1165 {
              tunnel: w1182 -> [w1189 _]
              tunnel: [w1188 w1193] -> w1171
              tunnel: w1170 -> [w1187 w1193]
              frame #0 {
                n342 = case shown="\"close-session\"" w1189 {
                  tunnel: [w1190 NTCP_Mixed_Mode_States."Ntcp.WaitForStart" ("NTCP MM States") NTCP_Mixed_Mode_States."Ntcp.Shutdown" ("NTCP MM States")] -> w1188
                  tunnel: w1187 -> [w1190 _ _]
                  frame #0 {
                  }
                  frame #1 {
                  }
                  frame #2 {
                  }
                }
              }
              frame #1 {
              }
            }
            n343 = Select(t=NTCP_Mixed_Mode_States."Ntcp.Shutdown", s=w1168, f=w1171) -> (s? t:f=w1169:T20)
            n344 = call <vilib>:"Merge Errors.vi"("error in 2 (no error)"=w1177, "error in 1 (no error)"=w1178) -> ("error out"=w1179:errorcluster)  [unwired: 5 in]
          }
          frame #4 {
            n345 = call "Start Or Stop.vi"("timeout"=w1201, "error in (no error)"=w1204, "AutoStart"=w1195, "MM Gui Updates In"=w1220, "MM Button Events In"=w1221) -> ("error out"=w1215:errorcluster, "Start or Stop"=w1217:T44, "MM Gui Updates Out"=w1218:refnum<queue>, "Button Events Out"=w1219:refnum<notifier>)  [unwired: 3 in]
            n346 = call "Monitor for NTCP Close.vi"("Skip"=Skip_NTCP_Close_Monitor."Skip Button Event", "timeout"=w1201, "error in (no error)"=w1204, "From NTCP In"=w1205) -> ("error out"=w1202:errorcluster, "From NTCP Out"=w1206:refnum<queue>, "Close Received"=w1198:bool)  [unwired: 4 in, 1 out]
            n347 = case shown="\"Accepted\"" w1217 {
              tunnel: [w1225 w1234 w1244 w1255] -> w1216
              tunnel: w1215 -> [w1224 w1230 w1240 w1254]
              tunnel: w1214 -> [w1225 w1234 w1244 w1253]
              tunnel: [w1224 w1227 w1237 w1252] -> w1213
              tunnel: [w1223 NTCP_Mixed_Mode_States."Ntcp.WaitForProposal" ("NTCP MM States") NTCP_Mixed_Mode_States."Ntcp.Shutdown" ("NTCP MM States") NTCP_Mixed_Mode_States."Ntcp.WaitForMclRamp" ("NTCP MM States")] -> w1199
              tunnel: w1212 -> [w1223 _ _ _]
              tunnel: w1211 -> [w1222 w1233 w1243 w1248]
              tunnel: w1210 -> [_ w1232 w1242 _]
              tunnel: [w1222 w1226 w1236 w1248] -> w1209
              frame #0 {
              }
              frame #1 {
                n348 = Bundle By Name(cluster=w1232, "NTCP commands"=NTCP_Commands."execute", "Accepted"=T24 FALSE) -> (w1231:T23)
                n349 = Enqueue Element(queue=w1233, element=w1231, error in (no error)=w1230) -> (queue out=w1226:refnum<queue>, error out=w1227:errorcluster)  [unwired: 1 in, 1 out]
              }
              frame #2 {
                n350 = Bundle By Name(cluster=w1242, "NTCP commands"=NTCP_Commands."execute", "Accepted"=T24 FALSE) -> (w1241:T23)
                n351 = Enqueue Element(queue=w1243, element=w1241, error in (no error)=w1240) -> (queue out=w1236:refnum<queue>, error out=w1237:errorcluster)  [unwired: 1 in, 1 out]
              }
              frame #3 {
                n352 = local read "Ramp Times"() -> (w1251:cluster{"Displacement":T15, "Force":T15})
                n353 = local read "Targets"() -> (w1250:T3[])
                n354 = call "Can Switch Control Types.vi"("Can Switch In"=FALSE, "DAO Actions"=DAO_Actions."Set") -> ()  [unwired: 9 in, 1 out]
                n355 = call "Send Mixed Mode Command.vi"("Targets"=w1250, "MCL Command In"=w1253, "Ramp Times"=w1251, "error in"=w1254) -> ("MCL Command Out"=w1255:refnum<queue>, "error out"=w1252:errorcluster)  [unwired: 1 in]
              }
            }
            n356 = call <vilib>:"Merge Errors.vi"("error in 3 (no error)"=w1213, "error in 2 (no error)"=w1202) -> ("error out"=w1203:errorcluster)  [unwired: 5 in]
            n357 = Select(t=NTCP_Mixed_Mode_States."Ntcp.Shutdown", s=w1198, f=w1199) -> (s? t:f=w1200:T20)
          }
          frame #5 {
            # "Note that the ramp does not stop\nif the connection is closed"
            n358 = call "Monitor for Stop.vi"("timeout"=w1266, "error in (no error)"=w1268, "Mixed Mode Commands In"=w1275, "MM Button Events In"=w1276) -> ("error out"=w1278:errorcluster, "Mixed Mode Commands Out"=w1274:refnum<queue>, "Stop Requests"=w1277:T45, "Button Events Out"=w1273:refnum<notifier>)  [unwired: 4 in]
            n359 = call "Monitor for NTCP Close.vi"("Skip"=Skip_NTCP_Close_Monitor."Skip Button Event", "timeout"=w1266, "error in (no error)"=w1268, "From NTCP In"=w1265) -> ("error out"=w1267:errorcluster, "From NTCP Out"=w1264:refnum<queue>, "Close Received"=w1263:bool)  [unwired: 4 in, 1 out]
            n360 = call "Done Or Abort.vi"("error in (no error)"=w1268, "timeout"=w1266, "MCL State In"=w1272) -> ("error out"=w1279:errorcluster, "MCL State"=w1280:T46, "MCL State Out"=w1271:refnum<queue>)  [unwired: 1 in]
            n361 = call <vilib>:"Merge Errors.vi"("error in 3 (no error)"=w1279, "error in 2 (no error)"=w1267, "error in 1 (no error)"=w1278) -> ("error out"=w1259:errorcluster)  [unwired: 4 in]
            n362 = call "Nctp Ramp Done.vi"("Close Received"=w1263, "MCL State In"=w1280, "error in"=w1259, "Stop Requests"=w1277, "MCL Cmd In"=w1261) -> ("error out"=w1256:errorcluster, "NTCP MM Finish State"=w1262:T20, "MCL Cmd Out"=w1260:refnum<queue>)  [unwired: 2 in]
          }
          frame #6 {
            n363 = call "Monitor for Stop.vi"("timeout"=w1293, "error in (no error)"=w1295, "Mixed Mode Commands In"=w1302, "MM Button Events In"=w1303) -> ("error out"=w1304:errorcluster, "Mixed Mode Commands Out"=w1301:refnum<queue>, "Stop Requests"=w1285:T45, "Button Events Out"=w1300:refnum<notifier>)  [unwired: 4 in]
            n364 = call "Monitor for NTCP Close.vi"("Skip"=Skip_NTCP_Close_Monitor."Skip Button Event", "timeout"=w1293, "error in (no error)"=w1295, "From NTCP In"=w1292) -> ("error out"=w1294:errorcluster, "From NTCP Out"=w1291:refnum<queue>, "Close Received"=w1283:bool)  [unwired: 4 in, 1 out]
            n365 = call "MCL Ramping.vi"("error in (no error)"=w1295, "timeout"=w1293, "MCL State In"=w1299) -> ("error out"=w1305:errorcluster, "Is Ramping?"=w1284:bool, "MCL State Out"=w1298:refnum<queue>)  [unwired: 1 in]
            n366 = call <vilib>:"Merge Errors.vi"("error in 3 (no error)"=w1305, "error in 2 (no error)"=w1294, "error in 1 (no error)"=w1304) -> ("error out"=w1288:errorcluster)  [unwired: 4 in]
            n367 = call "Nctp Ramp Running.vi"("Close Received"=w1283, "MCL Ramp Running?"=w1284, "error in"=w1288, "Stop Requests"=w1285, "MCL Cmd In"=w1286) -> ("error out"=w1281:errorcluster, "NTCP MM Finish State"=w1282:T20, "MCL Cmd Out"=w1287:refnum<queue>)  [unwired: 2 in]
          }
          frame #7 {
            # "Need to send an app event"
            n368 = Bundle By Name(cluster=w1315, "Command"=MM_Widget_Parameter_Changes."NTCP Link Off") -> (w1314:T30)
            n369 = Bundle By Name(cluster=w1329, "MM GUI Update Type"=Mixed_Mode_GUI_Update_Type."NTCP Server", "State"=FALSE) -> (w1326:T28)
            n370 = Send Notification(notification=w1314, notifier=w1319, error in (no error)=w1318) -> (notifier out=w1316:refnum<notifier>, error out=w1317:errorcluster)
            n371 = call "Can Switch Control Types.vi"("Can Switch In"=TRUE, "DAO Actions"=DAO_Actions."Set") -> ()  [unwired: 9 in, 1 out]
            n372 = Enqueue Element(queue=w1330, element=w1326, error in (no error)=w1317) -> (queue out=w1312:refnum<queue>, error out=w1310:errorcluster)  [unwired: 1 in, 1 out]
            n373 = call "Autos Off.vi"("error in"=w1310, "queue in"=w1312) -> ("error out"=w1309:errorcluster, "queue out"=w1311:refnum<queue>)  [unwired: 2 in]
          }
        }
      }
    }
    "NTCP MM States" <- w900
  }
  n374 = while {
    shift-right: [w1340] -> _
    shift-left: w2 -> [w1348]
    shift-right: [w1344] -> _
    shift-left: w32 -> [w1349]
    shift-right: [w1341] -> _
    shift-left: w17 -> [w1343]
    shift-right: [w1339] -> _
    shift-left: _ -> [w1338]
    tunnel: [w1336] -> w27
    shift-right: [w1331] -> _
    shift-left: w1 -> [w1332]
    stop <- w1336 stop-if-true
    # "Master Control Loop\nState Monitor"
    n375 = Dequeue Element(queue=w1349, timeout in ms (-1)=200, error in (no error)=w1348) -> (queue out=w1344:refnum<queue>, element=w1345:T9, timed out?=w1346:bool, error out=w1342:errorcluster)
    n376 = call "Fault List 2 Indicators.vi"("Use LBCB Selector"=FALSE) -> ("Forces"=w1333:bool, "Displacement"=w1334:bool)  [unwired: 8 in, 1 out]
    n377 = case shown="True" w1346 {
      tunnel: w1345 -> [w1352 _]
      tunnel: w1343 -> [w1361 w1396]
      tunnel: w1342 -> [w1351 w1395]
      tunnel: [w1360 w1396] -> w1341
      tunnel: [w1359 w1395] -> w1340
      tunnel: [w1355 w1397] -> w1339
      tunnel: w1338 -> [w1356 w1397]
      tunnel: w1332 -> [w1354 w1394]
      tunnel: [w1353 w1394] -> w1331
      frame #0 {
        n378 = Enqueue Element(queue=w1354, element=w1352, error in (no error)=w1351) -> (queue out=w1353:refnum<queue>, error out=w1350:errorcluster)  [unwired: 1 in, 1 out]
        n379 = case shown="\"Idle\"" w1352 {
          tunnel: [MCL_States."MCL Idle" ("notification") MCL_States."MCL Idle" ("notification") MCL_States."MCL Idle" ("notification") MCL_States."MCL Idle" ("notification") MCL_States."MCL Idle" ("notification") MCL_States."MCL Ramping" ("notification") MCL_States."MCL Ramping" ("notification") MCL_States."MCL Ramping" ("notification") MCL_States."MCL Ramping" ("notification") MCL_States."MCL Ramping" ("notification") MCL_States."MCL Ramping" ("notification") MCL_States."MCL Ramping" ("notification") MCL_States."MCL Ramping" ("notification") MCL_States."MCL Ramping" ("notification") MCL_States."MCL Ramping" ("notification") MCL_States."MCL Ramping" ("notification") MCL_States."MCL Ramping" ("notification") MCL_States."MCL Holding" ("notification") MCL_States."MCL Holding" ("notification") MCL_States."MCL Holding" ("notification") MCL_States."MCL Holding" ("notification") MCL_States."MCL Done" ("notification") MCL_States."MCL Aborting" ("notification") MCL_States."MCL Done" ("notification") MCL_States."MCL Idle" ("notification")] -> w1355
          frame #0 {
          }
          frame #1 {
          }
          frame #2 {
          }
          frame #3 {
          }
          frame #4 {
          }
          frame #5 {
          }
          frame #6 {
          }
          frame #7 {
          }
          frame #8 {
          }
          frame #9 {
          }
          frame #10 {
          }
          frame #11 {
          }
          frame #12 {
          }
          frame #13 {
          }
          frame #14 {
          }
          frame #15 {
          }
          frame #16 {
          }
          frame #17 {
          }
          frame #18 {
          }
          frame #19 {
          }
          frame #20 {
          }
          frame #21 {
          }
          frame #22 {
          }
          frame #23 {
          }
          frame #24 {
          }
        }
        n380 = call "States 2 Leds.vi"("MixedModeStates"=w1352) -> ("Mixed Mode State Display"=w1358:T22)  [unwired: 10 in]
        n381 = local write "Mixed Mode State Display"(w1358) -> ()
        n382 = Not Equal?(x=w1355, y=w1356) -> (x != y?=w1357:bool)
        n383 = case shown="True" w1357 {
          tunnel: w1361 -> [w1363 w1368]
          tunnel: w1350 -> [w1362 w1367]
          tunnel: [w1363 w1366] -> w1360
          tunnel: [w1362 w1365] -> w1359
          tunnel: w1355 -> [_ w1364]
          frame #0 {
          }
          frame #1 {
            n384 = Enqueue Element(queue=w1368, element=w1364, error in (no error)=w1367) -> (queue out=w1366:refnum<queue>, error out=w1365:errorcluster)  [unwired: 1 in, 1 out]
          }
        }
        n385 = local write "MCL States"(w1355) -> ()
      }
      frame #1 {
      }
    }
    n386 = local write "Displacement Limit"(w1334) -> ()
    n387 = local write "Force Limit"(w1333) -> ()
    n388 = local read "Button States"() -> (w1337:T12)
    n389 = Unbundle By Name(w1337) -> ("Exit Requested"=w1336:bool)
  }
  n390 = Compound Arithmetic op=AND(w44, w43, w40, w28, w24, w27, w23, w16) -> (w51:bool)
  n391 = Not(x=w51) -> (.not. x?=w50:bool)
  n392 = flat-sequence {
    tunnel: w50 -> [w1400]
    tunnel: [w1400] -> w49
    frame #0 {
      n393 = control-ref of="This VI"() -> (w1399:refnum<vi>)
      n394 = disable-structure shown="Disabled" {
        disable-tunnel: w1399 -> [w1402 _]
        disable-tunnel: FALSE ("Front Panel Window:Open") -> [w1401 _]
        frame #0 {
          n395 = property class="VI"(reference=w1402, "Front Panel.Open"=w1401) -> ()  [unwired: 1 in, 2 out]
        }
        frame #1 {
        }
      }
    }
  }
  n396 = local write "App Stop"(w49) -> ()
